vi "validate_experiment_pharmaBot_v0.06.vi"(0 "ExperimentOptionsCluster":T1, 1 "Open Tip?":bool, 4 "Graph cluster":T4, 7 "error in":errorcluster, 8 "which manipulator":T6(ring), 9 "common cluster":T8, 14 "controls array":refnum<vi>[](array[refnum]), 15 "individual controls in":T7, 17 "data in":T5={"daq_ao 1"="Dev1/ao0", "daq_ai 1"="Dev1/ai0", "experiment day folder"=path "D:/DATA/8-27-15 save func testing/test.lvm", "Multiclamp init error"=0, "Multiclamp Handle Out"=0, "sampling rate (Hz)"=10000, "trial name"=""}) -> (16 "control array out":refnum<vi>[](array[refnum]), 20 "ValidationWaveform":waveform(dbl)[](array[waveform]), 21 "protocol waveform":waveform(dbl)(graph), 22 "ValidationResults":waveform(dbl)[][](array[waveform]), 23 "ValidationPos1":T3(array[ring]), 24 "protocol response":waveform(dbl)[](graph), 25 "ValidationPos2":T3(array[ring]), 26 "ValidationOutputCluster":T2(array[cluster]), 27 "error out":errorcluster)   [LabVIEW 2019]
uses:
  pipette cleaning/pressure box/cleaning_soft/controls/actuator_type.ctl
  pipette cleaning/pressure box/cleaning_soft/controls/actuator_cluster.ctl
  machine_vision/coordinate model vis/transform_properties_actuators.ctl
  machine_vision/controls/transform_cluster_actuator.ctl
  controls/NH_method.ctl
  pipette cleaning/pressure box/cleaning_soft/controls/pressure_box_type.ctl
  pipette cleaning/pressure box/cleaning_soft/controls/pressure_box_control.ctl
  multipatch/controls/multipatch_common_controls_v4.ctl
  controls/memtest_def.ctl
  multipatch/controls/multipatch_individual_controls_v5.ctl
  Controls/Data.ctl
panel:
  out "curMJumpAlreadyValid":bool
  out "Jump Pos o-C":bool
  out "Jump Pos C-o":bool
  out "Jump Pos C-B":bool
  out "Jump Pos B-C":bool
  out "Jump Pos B-A":bool
  out "Jump Pos A-B":bool
  out "Jump Pos A-o":bool
  out "Jump Pos o-A":bool
  out "Pos C":bool
  out "Pos B":bool
  out "Pos A":bool
  out "Experiment Safe":bool
  out "Jumper Safe":bool
  # "already validated?"
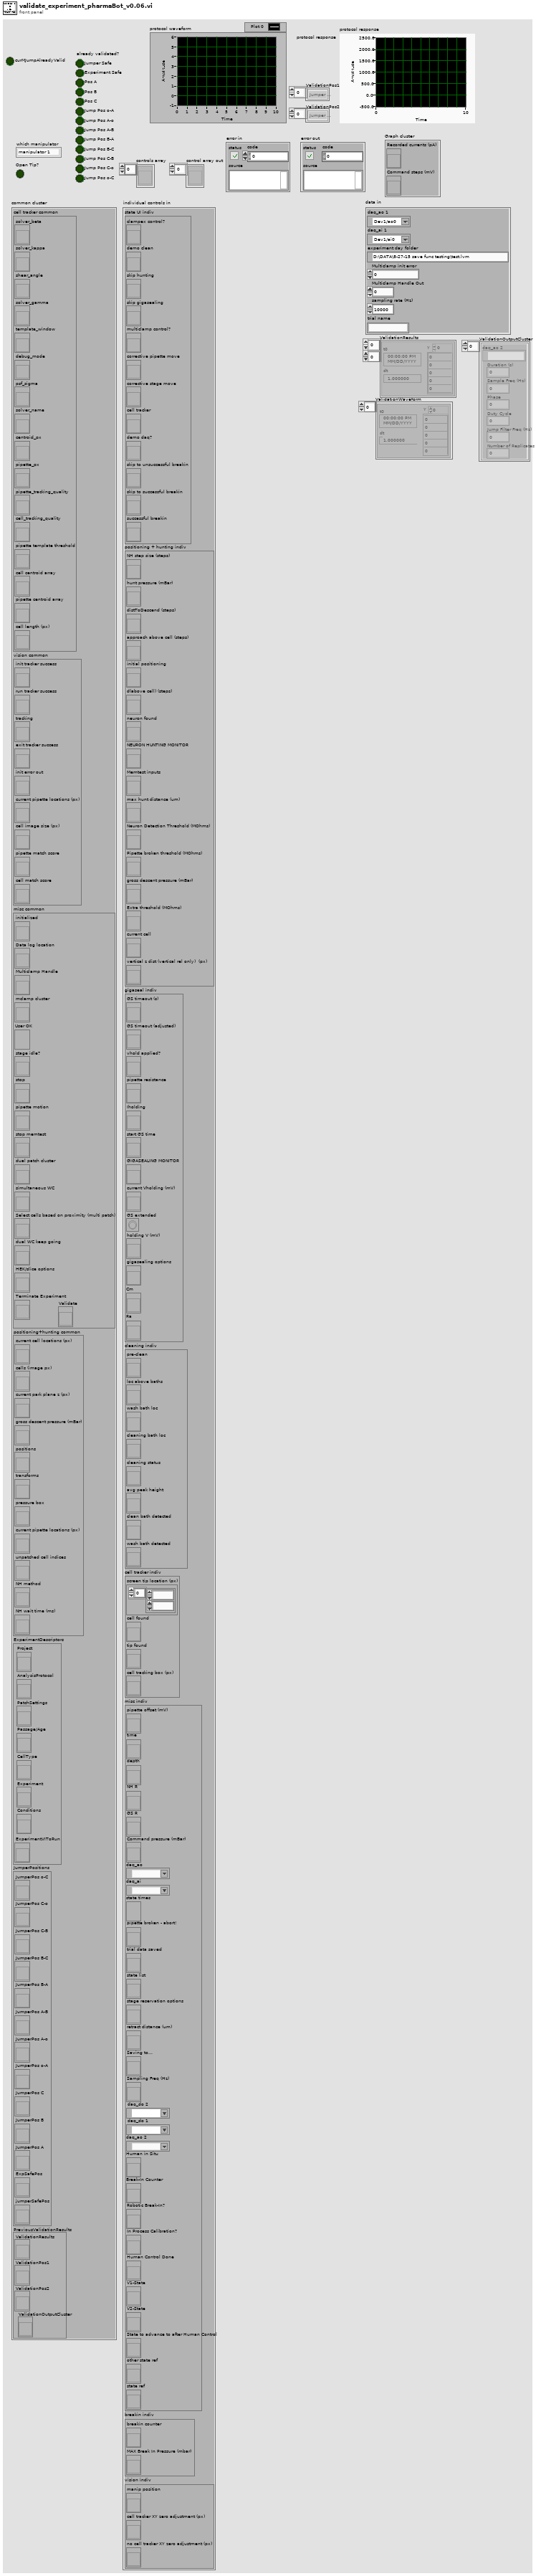
[diagram p1: front panel]
types:
  T1 = cluster{"How Many Experimental Phases?":refnum<vi>, "PhaseA Cluster":cluster{"Phase Experiment Option":refnum<vi>, "Paired Pulse":refnum<vi>, "Jump Train":refnum<vi>, "Voltage Ramp":refnum<vi>, "Voltage Step":refnum<vi>, "Solution Change":refnum<vi>, "Single Jump":refnum<vi>, "Single Manip Jump":refnum<vi>, "Gap Free":refnum<vi>, "Multi Manip Jump":refnum<vi>, "Voltage Pulse":refnum<vi>, "Current Pulse":refnum<vi>, "Current Ramp":refnum<vi>, "Gap Free Iclamp":refnum<vi>}, "PhaseB Cluster":cluster{"Phase Experiment Option":refnum<vi>, "Paired Pulse":refnum<vi>, "Jump Train":refnum<vi>, "Voltage Ramp":refnum<vi>, "Voltage Step":refnum<vi>, "Solution Change":refnum<vi>, "Single Jump":refnum<vi>, "Single Manip Jump":refnum<vi>, "Gap Free":refnum<vi>, "Multi Manip Jump":refnum<vi>, "Voltage Pulse":refnum<vi>, "Current Pulse":refnum<vi>, "Current Ramp":refnum<vi>, "Gap Free Iclamp":refnum<vi>}, "PhaseC Cluster":cluster{"Phase Experiment Option":refnum<vi>, "Paired Pulse":refnum<vi>, "Jump Train":refnum<vi>, "Voltage Ramp":refnum<vi>, "Voltage Step":refnum<vi>, "Solution Change":refnum<vi>, "Single Jump":refnum<vi>, "Single Manip Jump":refnum<vi>, "Gap Free":refnum<vi>, "Multi Manip Jump":refnum<vi>, "Voltage Pulse":refnum<vi>, "Current Pulse":refnum<vi>, "Current Ramp":refnum<vi>, "Gap Free Iclamp":refnum<vi>}, "PhaseD Cluster":cluster{"Phase Experiment Option":refnum<vi>, "Paired Pulse":refnum<vi>, "Jump Train":refnum<vi>, "Voltage Ramp":refnum<vi>, "Voltage Step":refnum<vi>, "Solution Change":refnum<vi>, "Single Jump":refnum<vi>, "Single Manip Jump":refnum<vi>, "Gap Free":refnum<vi>, "Multi Manip Jump":refnum<vi>, "Voltage Pulse":refnum<vi>, "Current Pulse":refnum<vi>, "Current Ramp":refnum<vi>, "Gap Free Iclamp":refnum<vi>}, "PhaseE Cluster":cluster{"Phase Experiment Option":refnum<vi>, "Paired Pulse":refnum<vi>, "Jump Train":refnum<vi>, "Voltage Ramp":refnum<vi>, "Voltage Step":refnum<vi>, "Solution Change":refnum<vi>, "Single Jump":refnum<vi>, "Single Manip Jump":refnum<vi>, "Gap Free":refnum<vi>, "Multi Manip Jump":refnum<vi>, "Voltage Pulse":refnum<vi>, "Current Pulse":refnum<vi>, "Current Ramp":refnum<vi>, "Gap Free Iclamp":refnum<vi>}, "PhaseF Cluster":cluster{"Phase Experiment Option":refnum<vi>, "Paired Pulse":refnum<vi>, "Jump Train":refnum<vi>, "Voltage Ramp":refnum<vi>, "Voltage Step":refnum<vi>, "Solution Change":refnum<vi>, "Single Jump":refnum<vi>, "Single Manip Jump":refnum<vi>, "Gap Free":refnum<vi>, "Multi Manip Jump":refnum<vi>, "Voltage Pulse":refnum<vi>, "Current Pulse":refnum<vi>, "Current Ramp":refnum<vi>, "Gap Free Iclamp":refnum<vi>}, "time to wait for solution change (min)":refnum<vi>, "valve Time Cluster":cluster{"time of Last V1 Change":refnum<vi>, "time of Last V2 Change":refnum<vi>, "time of Last V3 Change":refnum<vi>}, "PhaseG Cluster":cluster{"Phase Experiment Option":refnum<vi>, "Paired Pulse":refnum<vi>, "Jump Train":refnum<vi>, "Voltage Ramp":refnum<vi>, "Voltage Step":refnum<vi>, "Solution Change":refnum<vi>, "Single Jump":refnum<vi>, "Single Manip Jump":refnum<vi>, "Gap Free":refnum<vi>, "Multi Manip Jump":refnum<vi>, "Voltage Pulse":refnum<vi>, "Current Pulse":refnum<vi>, "Current Ramp":refnum<vi>, "Gap Free Iclamp":refnum<vi>}, "PhaseH Cluster":cluster{"Phase Experiment Option":refnum<vi>, "Paired Pulse":refnum<vi>, "Jump Train":refnum<vi>, "Voltage Ramp":refnum<vi>, "Voltage Step":refnum<vi>, "Solution Change":refnum<vi>, "Single Jump":refnum<vi>, "Single Manip Jump":refnum<vi>, "Gap Free":refnum<vi>, "Multi Manip Jump":refnum<vi>, "Voltage Pulse":refnum<vi>, "Current Pulse":refnum<vi>, "Current Ramp":refnum<vi>, "Gap Free Iclamp":refnum<vi>}, "PhaseI Cluster":cluster{"Phase Experiment Option":refnum<vi>, "Paired Pulse":refnum<vi>, "Jump Train":refnum<vi>, "Voltage Ramp":refnum<vi>, "Voltage Step":refnum<vi>, "Solution Change":refnum<vi>, "Single Jump":refnum<vi>, "Single Manip Jump":refnum<vi>, "Gap Free":refnum<vi>, "Multi Manip Jump":refnum<vi>, "Voltage Pulse":refnum<vi>, "Current Pulse":refnum<vi>, "Current Ramp":refnum<vi>, "Gap Free Iclamp":refnum<vi>}, "PhaseJ Cluster":cluster{"Phase Experiment Option":refnum<vi>, "Paired Pulse":refnum<vi>, "Jump Train":refnum<vi>, "Voltage Ramp":refnum<vi>, "Voltage Step":refnum<vi>, "Solution Change":refnum<vi>, "Single Jump":refnum<vi>, "Single Manip Jump":refnum<vi>, "Gap Free":refnum<vi>, "Multi Manip Jump":refnum<vi>, "Voltage Pulse":refnum<vi>, "Current Pulse":refnum<vi>, "Current Ramp":refnum<vi>, "Gap Free Iclamp":refnum<vi>}, "PhaseK Cluster":cluster{"Phase Experiment Option":refnum<vi>, "Paired Pulse":refnum<vi>, "Jump Train":refnum<vi>, "Voltage Ramp":refnum<vi>, "Voltage Step":refnum<vi>, "Solution Change":refnum<vi>, "Single Jump":refnum<vi>, "Single Manip Jump":refnum<vi>, "Gap Free":refnum<vi>, "Multi Manip Jump":refnum<vi>, "Voltage Pulse":refnum<vi>, "Current Pulse":refnum<vi>, "Current Ramp":refnum<vi>, "Gap Free Iclamp":refnum<vi>}, "PhaseL Cluster":cluster{"Phase Experiment Option":refnum<vi>, "Paired Pulse":refnum<vi>, "Jump Train":refnum<vi>, "Voltage Ramp":refnum<vi>, "Voltage Step":refnum<vi>, "Solution Change":refnum<vi>, "Single Jump":refnum<vi>, "Single Manip Jump":refnum<vi>, "Gap Free":refnum<vi>, "Multi Manip Jump":refnum<vi>, "Voltage Pulse":refnum<vi>, "Current Pulse":refnum<vi>, "Current Ramp":refnum<vi>, "Gap Free Iclamp":refnum<vi>}, "PhaseStatusCluster":cluster{"Phase A Done":refnum<vi>, "Phase B Done":refnum<vi>, "Phase C Done":refnum<vi>, "Phase D Done":refnum<vi>, "Phase E Done":refnum<vi>, "Phase F Done":refnum<vi>, "Phase G Done":refnum<vi>, "Phase H Done":refnum<vi>, "Phase I Done":refnum<vi>, "Phase J Done":refnum<vi>, "Phase K Done":refnum<vi>, "Phase L Done":refnum<vi>}}
  T2 = cluster{"daq_ao 2":tag, "Duration (s)":dbl, "Sample Freq (Hz)":dbl, "Phase":dbl, "Duty Cycle":dbl, "Jump Filter Freq (Hz)":dbl, "Number of Replicates":i16}[]
  T3 = enum16{"Jumper Safe Position", "Experiment Safe Position", "Jumper Position A", "Jumper Position B", "Jumper Position C", "Jumper Position o-A", "Jumper Position A-o", "Jumper Position A-B", "Jumper Position B-A", "Jumper Position B-C", "Jumper Position C-B", "Jumper Position C-o", "Jumper Position o-C"}[]
  T4 = cluster{"Recorded currents (pA)":refnum<vi>, "Command steps (mV)":refnum<vi>}
  T5 = typedef "Data.ctl" = cluster{"daq_ao 1":tag, "daq_ai 1":tag, "experiment day folder":path, "Multiclamp init error":i32, "Multiclamp Handle Out":u32, "sampling rate (Hz)":i32, "trial name":string}
  T6 = enum16{"manipulator 1", "manipulator 2", "manipulator 3", "manipulator 4"}
  T7 = typedef "multipatch_individual_controls_v5.ctl" = cluster{"state UI indiv":cluster{"clampex control?":refnum<vi>, "demo clean":refnum<vi>, "skip hunting":refnum<vi>, "skip gigasealing":refnum<vi>, "multiclamp control?":refnum<vi>, "corrective pipette move":refnum<vi>, "corrective stage move":refnum<vi>, "cell tracker":refnum<vi>, "demo daq?":refnum<vi>, "skip to unsuccessful breakin":refnum<vi>, "skip to successful breakin":refnum<vi>, "successful breakin":refnum<vi>}, "positioning + hunting indiv":cluster{"NH step size (steps)":refnum<vi>, "hunt pressure (mBar)":refnum<vi>, "distToDescend (steps)":refnum<vi>, "approach above cell (steps)":refnum<vi>, "initial positioning":refnum<vi>, "d(above cell) (steps)":refnum<vi>, "neuron found":refnum<vi>, "NEURON HUNTING MONITOR":refnum<vi>, "Memtest inputs":refnum<vi>, "max hunt distance (um)":refnum<vi>, "Neuron Detection Threshold (MOhms)":refnum<vi>, "Pipette broken threshold (MOhms)":refnum<vi>, "gross descent pressure (mBar)":refnum<vi>, "Extra threshold (MOhms)":refnum<vi>, "current cell":refnum<vi>, "vertical z dist (vertical rel only)  (px)":refnum<vi>}, "gigaseal indiv":cluster{"GS timeout (s)":refnum<vi>, "GS timeout (adjusted)":refnum<vi>, "vhold applied?":refnum<vi>, "pipette resistance":refnum<vi>, "Iholding":refnum<vi>, "start GS time":refnum<vi>, "GIGASEALING MONITOR":refnum<vi>, "current Vholding (mV)":refnum<vi>, "GS extended":refnum<vi>, "holding V (mV)":refnum<vi>, "gigasealing options":refnum<vi>, "Cm":refnum<vi>, "Ra ":refnum<vi>}, "cleaning indiv":cluster{"pre-clean":refnum<vi>, "loc above baths":refnum<vi>, "wash bath loc":refnum<vi>, "cleaning bath loc":refnum<vi>, "cleaning status":refnum<vi>, "avg peak height":refnum<vi>, "clean bath detected":refnum<vi>, "wash bath detected":refnum<vi>}, "cell tracker indiv":cluster{"screen tip location (px)":refnum<vi>, "cell found":refnum<vi>, "tip found":refnum<vi>, "cell tracking box (px)":refnum<vi>}, "misc indiv":cluster{"pipette offset (mV)":refnum<vi>, "time":refnum<vi>, "depth":refnum<vi>, "NH R":refnum<vi>, "GS R":refnum<vi>, "Command pressure (mBar)":refnum<vi>, "daq_ao":tag, "daq_ai":tag, "state times":refnum<vi>, "pipette broken - abort!":refnum<vi>, "trial data saved":refnum<vi>, "state list":refnum<vi>, "stage reservation options":refnum<vi>, "retract distance (um)":refnum<vi>, "Saving to...":refnum<vi>, "Sampling Freq (Hz)":refnum<vi>, "daq_do 2":tag, "daq_do 1":tag, "daq_ao 2":tag, "Human in Situ":refnum<vi>, "Break-In Counter":refnum<vi>, "Robotic Break-In?":refnum<vi>, "In Process Calibration?":refnum<vi>, "Human Control Done":refnum<vi>, "V1-State":refnum<vi>, "V2-State":refnum<vi>, "State to advance to after Human Control":refnum<vi>, "other state ref":refnum<vi>, "state ref":refnum<vi>}, "breakin indiv":cluster{"breakin counter":refnum<vi>, "MAX Break In Pressure (mbar)":refnum<vi>}, "vision indiv":cluster{"manip position":refnum<vi>, "cell tracker XY zero adjustment (px)":refnum<vi>, "no cell tracker XY zero adjustment (px)":refnum<vi>}}
  T8 = typedef "multipatch_common_controls_v4.ctl" = cluster{"cell tracker common":cluster{"solver_beta":refnum<vi>, "solver_kappa":refnum<vi>, "shear_angle":refnum<vi>, "solver_gamma":refnum<vi>, "template_window":refnum<vi>, "debug_mode":refnum<vi>, "psf_sigma":refnum<vi>, "solver_name":refnum<vi>, "centroid_px":refnum<vi>, "pipette_px":refnum<vi>, "pipette_tracking_quality":refnum<vi>, "cell_tracking_quality":refnum<vi>, "pipette template threshold":refnum<vi>, "cell centroid array":refnum<vi>, "pipette centroid array":refnum<vi>, "cell length (px)":refnum<vi>}, "vision common":cluster{"init tracker success":refnum<vi>, "run tracker success":refnum<vi>, "tracking":refnum<vi>, "exit tracker success":refnum<vi>, "init error out":refnum<vi>, "current pipette locations (px)":refnum<vi>, "cell image size (px)":refnum<vi>, "pipette match score":refnum<vi>, "cell match score":refnum<vi>}, "misc common":cluster{"initialized":refnum<vi>, "Data log location":refnum<vi>, "Multiclamp Handle":refnum<vi>, "mclamp cluster":refnum<vi>, "User OK":refnum<vi>, "stage idle?":refnum<vi>, "stop":refnum<vi>, "pipette motion":refnum<vi>, "stop memtest":refnum<vi>, "dual patch cluster":refnum<vi>, "simultaneous WC":refnum<vi>, "Select cells based on proximity (multi patch)":refnum<vi>, "dual WC keep going":refnum<vi>, "HEK/slice options":refnum<vi>, "Terminate Experiment":refnum<vi>, "Validate":refnum<vi>}, "positioning+hunting common":cluster{"current cell locations (px)":refnum<vi>, "cells (image px)":refnum<vi>, "current park plane z (px)":refnum<vi>, "gross descent pressure (mBar)":refnum<vi>, "positions":refnum<vi>, "transforms":refnum<vi>, "pressure box":refnum<vi>, "current pipette locations (px)":refnum<vi>, "unpatched cell indices":refnum<vi>, "NH method":refnum<vi>, "NH wait time (ms)":refnum<vi>}, "ExperimentDescriptors":cluster{"Project":refnum<vi>, "AnalysisProtocol":refnum<vi>, "PatchSettings":refnum<vi>, "Passage/Age":refnum<vi>, "CellType":refnum<vi>, "Experiment":refnum<vi>, "Conditions":refnum<vi>, "ExperimentVIToRun":refnum<vi>}, "JumperPositions":cluster{"JumperPos o-C":refnum<vi>, "JumperPos C-o":refnum<vi>, "JumperPos C-B":refnum<vi>, "JumperPos B-C":refnum<vi>, "JumperPos B-A":refnum<vi>, "JumperPos A-B":refnum<vi>, "JumperPos A-o":refnum<vi>, "JumperPos o-A":refnum<vi>, "JumperPos C":refnum<vi>, "JumperPos B":refnum<vi>, "JumperPos A":refnum<vi>, "ExpSafePos":refnum<vi>, "jumperSafePos":refnum<vi>}, "PreviousValidationResults":cluster{"ValidationResults":refnum<vi>, "ValidationPos1":refnum<vi>, "ValidationPos2":refnum<vi>, "ValidationOutputCluster":refnum<vi>}}
  T9 = cluster{"time of Last V1 Change":refnum<vi>, "time of Last V2 Change":refnum<vi>, "time of Last V3 Change":refnum<vi>}
  T10 = typedef "pressure_box_control.ctl" = cluster{"Pressure box COM":refnum<visa-resource-name>, "pressure box type":T11, "High pos pressure (mBar)":dbl, "Low pos pressure (mBar)":dbl, "Vacuum pressure (mBar)":dbl, "calibration":enum16{"PA_vacPump", "PA_venturi", "Neuromatics", "ilyaRig", "mightenRig"}}
  T11 = typedef "pressure_box_type.ctl" = enum16{"Neuromatics", "ProportionAir", "Demo box", "N-ProportionAir"}
  T12 = cluster{"daq_ao 2":tag, "Duration (s)":dbl, "Sample Freq (Hz)":dbl, "Phase":dbl, "Duty Cycle":dbl, "Jump Filter Freq (Hz)":dbl, "Number of Replicates":i16}
  T13 = enum16{"Jumper Safe Position", "Experiment Safe Position", "Jumper Position A", "Jumper Position B", "Jumper Position C", "Jumper Position o-A", "Jumper Position A-o", "Jumper Position A-B", "Jumper Position B-A", "Jumper Position B-C", "Jumper Position C-B", "Jumper Position C-o", "Jumper Position o-C"}
  T14 = cluster{u32, string, i32, u32, u32, u32, "arg1":i32}
  T15 = cluster{"Phase Experiment Option":refnum<vi>, "Paired Pulse":refnum<vi>, "Jump Train":refnum<vi>, "Voltage Ramp":refnum<vi>, "Voltage Step":refnum<vi>, "Solution Change":refnum<vi>, "Single Jump":refnum<vi>, "Single Manip Jump":refnum<vi>, "Gap Free":refnum<vi>, "Multi Manip Jump":refnum<vi>, "Voltage Pulse":refnum<vi>, "Current Pulse":refnum<vi>, "Current Ramp":refnum<vi>, "Gap Free Iclamp":refnum<vi>}
  T16 = cluster{"Which Position to use for Experiment":enum16{"Jumper Safe Position", "Experiment Safe Position", "Jumper Position A", "Jumper Position B", "Jumper Position C", "Jumper Position o-A", "Jumper Position A-o", "Jumper Position A-B", "Jumper Position B-A", "Jumper Position B-C", "Jumper Position C-B", "Jumper Position C-o", "Jumper Position o-C", "Don't Move"}, "Start Position (N)":string, "Jump Position (m)":string, "Duration (s)":dbl, "Delay (s)":dbl, "Pulse Width (s)":dbl, "Valve 1 Position":i16, "Valve 2 Position":i16, "Replicates":dbl, "Vholding (mV)":dbl, "Valve 3 Position":i16, "valve 1 used now?":bool, "valve 2 used now?":bool, "valve 3 used now? ":bool, "protocol Preview":waveform(dbl)[]}
  T17 = enum16{"Jumper Safe Position", "Experiment Safe Position", "Jumper Position A", "Jumper Position B", "Jumper Position C", "Jumper Position o-A", "Jumper Position A-o", "Jumper Position A-B", "Jumper Position B-A", "Jumper Position B-C", "Jumper Position C-B", "Jumper Position C-o", "Jumper Position o-C", "Don't Move"}
  T18 = cluster{"Which Position to use for Experiment":enum16{"Jumper Safe Position", "Experiment Safe Position", "Jumper Position A", "Jumper Position B", "Jumper Position C", "Jumper Position o-A", "Jumper Position A-o", "Jumper Position A-B", "Jumper Position B-A", "Jumper Position B-C", "Jumper Position C-B", "Jumper Position C-o", "Jumper Position o-C", "Don't Move"}, "Duration (s)":dbl, "Delay (s)":dbl, "Pulse Width (s)":dbl, "Which Valve to Change?":i16, "Valve Jump Position":i16, "Replicates":dbl, "Vholding (mV)":dbl, "valve 1 used now?":bool, "valve 2 used now?":bool, "valve 3 used now? ":bool, "Valve 1 Position":i16, "Valve 2 Position":i16, "Valve 3 Position":i16, "protocol Preview":waveform(dbl)[]}
  T19 = cluster{"Which Position to use for Experiment":enum16{"Jumper Safe Position", "Experiment Safe Position", "Jumper Position A", "Jumper Position B", "Jumper Position C", "Jumper Position o-A", "Jumper Position A-o", "Jumper Position A-B", "Jumper Position B-A", "Jumper Position B-C", "Jumper Position C-B", "Jumper Position C-o", "Jumper Position o-C", "Don't Move"}, "Duration (s)":dbl, "Delay (s)":dbl, "Step Width (s)":dbl, "Voltage Start (mV)":dbl, "Voltage Step (mV)":dbl, "Replicates":dbl, "Voltage End (mV)":dbl, "Number of Step":dbl, "Vholding (mV)":dbl, "Valve 1 Position":i16, "Valve 2 Position":i16, "Valve 3 Position":i16, "valve 1 used now?":bool, "valve 2 used now?":bool, "valve 3 used now? ":bool, "Total Step Time (s)":dbl, "Maintain Final Voltage until end?":bool, "protocol Preview":waveform(dbl)[]}
  T20 = cluster{"Which Position to use for Experiment":enum16{"Jumper Safe Position", "Experiment Safe Position", "Jumper Position A", "Jumper Position B", "Jumper Position C", "Jumper Position o-A", "Jumper Position A-o", "Jumper Position A-B", "Jumper Position B-A", "Jumper Position B-C", "Jumper Position C-B", "Jumper Position C-o", "Jumper Position o-C", "Don't Move"}, "Duration (s)":dbl, "Delay (s)":dbl, "Ramp Slope (mV/s)":dbl, "Voltage Start (mV)":dbl, "Replicates":dbl, "Voltage End (mV)":dbl, "Ramp Duration (s)":dbl, "Vholding (mV)":dbl, "Valve 1 Position":i16, "Valve 2 Position":i16, "Valve 3 Position":i16, "valve 1 used now?":bool, "valve 2 used now?":bool, "valve 3 used now? ":bool, "Maintain Final Voltage until end?":bool, "protocol Preview":waveform(dbl)[]}
  T21 = cluster{"Which Position to use for Experiment":enum16{"Jumper Safe Position", "Experiment Safe Position", "Jumper Position A", "Jumper Position B", "Jumper Position C", "Jumper Position o-A", "Jumper Position A-o", "Jumper Position A-B", "Jumper Position B-A", "Jumper Position B-C", "Jumper Position C-B", "Jumper Position C-o", "Jumper Position o-C", "Don't Move"}, "Start Position (N)":string, "Jump Position (m)":string, "Duration (s)":dbl, "Delay (s)":dbl, "Pulse Width (s)":dbl, "Valve 1 Position":i16, "Valve 2 Position":i16, "Replicates":dbl, "Pulse Period (s)":dbl, "Vholding (mV)":dbl, "Number of Pulses":dbl, "valve 1 used now?":bool, "valve 2 used now?":bool, "valve 3 used now? ":bool, "Valve 3 Position":i16, "protocol Preview":waveform(dbl)[]}
  T22 = cluster{"Which Position to use for Experiment":enum16{"Jumper Safe Position", "Experiment Safe Position", "Jumper Position A", "Jumper Position B", "Jumper Position C", "Jumper Position o-A", "Jumper Position A-o", "Jumper Position A-B", "Jumper Position B-A", "Jumper Position B-C", "Jumper Position C-B", "Jumper Position C-o", "Jumper Position o-C", "Don't Move"}, "Start Position (N)":string, "Jump Position (m)":string, "Duration (s)":dbl, "Delay (s)":dbl, "Pulse Width (s)":dbl, "Replicates":dbl, "Pulse Delay (s)":dbl, "Pulse Delta Delay (s)":dbl, "Vholding (mV)":dbl, "Valve 1 Position":i16, "Valve 2 Position":i16, "valve 1 used now?":bool, "valve 2 used now?":bool, "valve 3 used now? ":bool, "Valve 3 Position":i16, "protocol Preview":waveform(dbl)[]}
  T23 = cluster{"Start Position (N)":enum16{"Jumper Safe Position", "Experiment Safe Position", "Jumper Position A", "Jumper Position B", "Jumper Position C", "Jumper Position o-A", "Jumper Position A-o", "Jumper Position A-B", "Jumper Position B-A", "Jumper Position B-C", "Jumper Position C-B", "Jumper Position C-o", "Jumper Position o-C", "Don't Move"}, "Duration (s)":dbl, "Delay (s)":dbl, "Pulse Width (s)":dbl, "Valve 1 Position":i16, "Valve 2 Position":i16, "Replicates":dbl, "Jump Position (m)":enum16{"Jumper Safe Position", "Experiment Safe Position", "Jumper Position A", "Jumper Position B", "Jumper Position C", "Jumper Position o-A", "Jumper Position A-o", "Jumper Position A-B", "Jumper Position B-A", "Jumper Position B-C", "Jumper Position C-B", "Jumper Position C-o", "Jumper Position o-C", "Don't Move"}, "Vholding (mV)":dbl, "Valve 3 Position":i16, "valve 1 used now?":bool, "valve 2 used now?":bool, "valve 3 used now? ":bool, "protocol Preview":waveform(dbl)[]}
  T24 = enum16{"Jumper Safe Position", "Experiment Safe Position", "Jumper Position A", "Jumper Position B", "Jumper Position C", "Jumper Position o-A", "Jumper Position A-o", "Jumper Position A-B", "Jumper Position B-A", "Jumper Position B-C", "Jumper Position C-B", "Jumper Position C-o", "Jumper Position o-C", "Don't Move"}[]
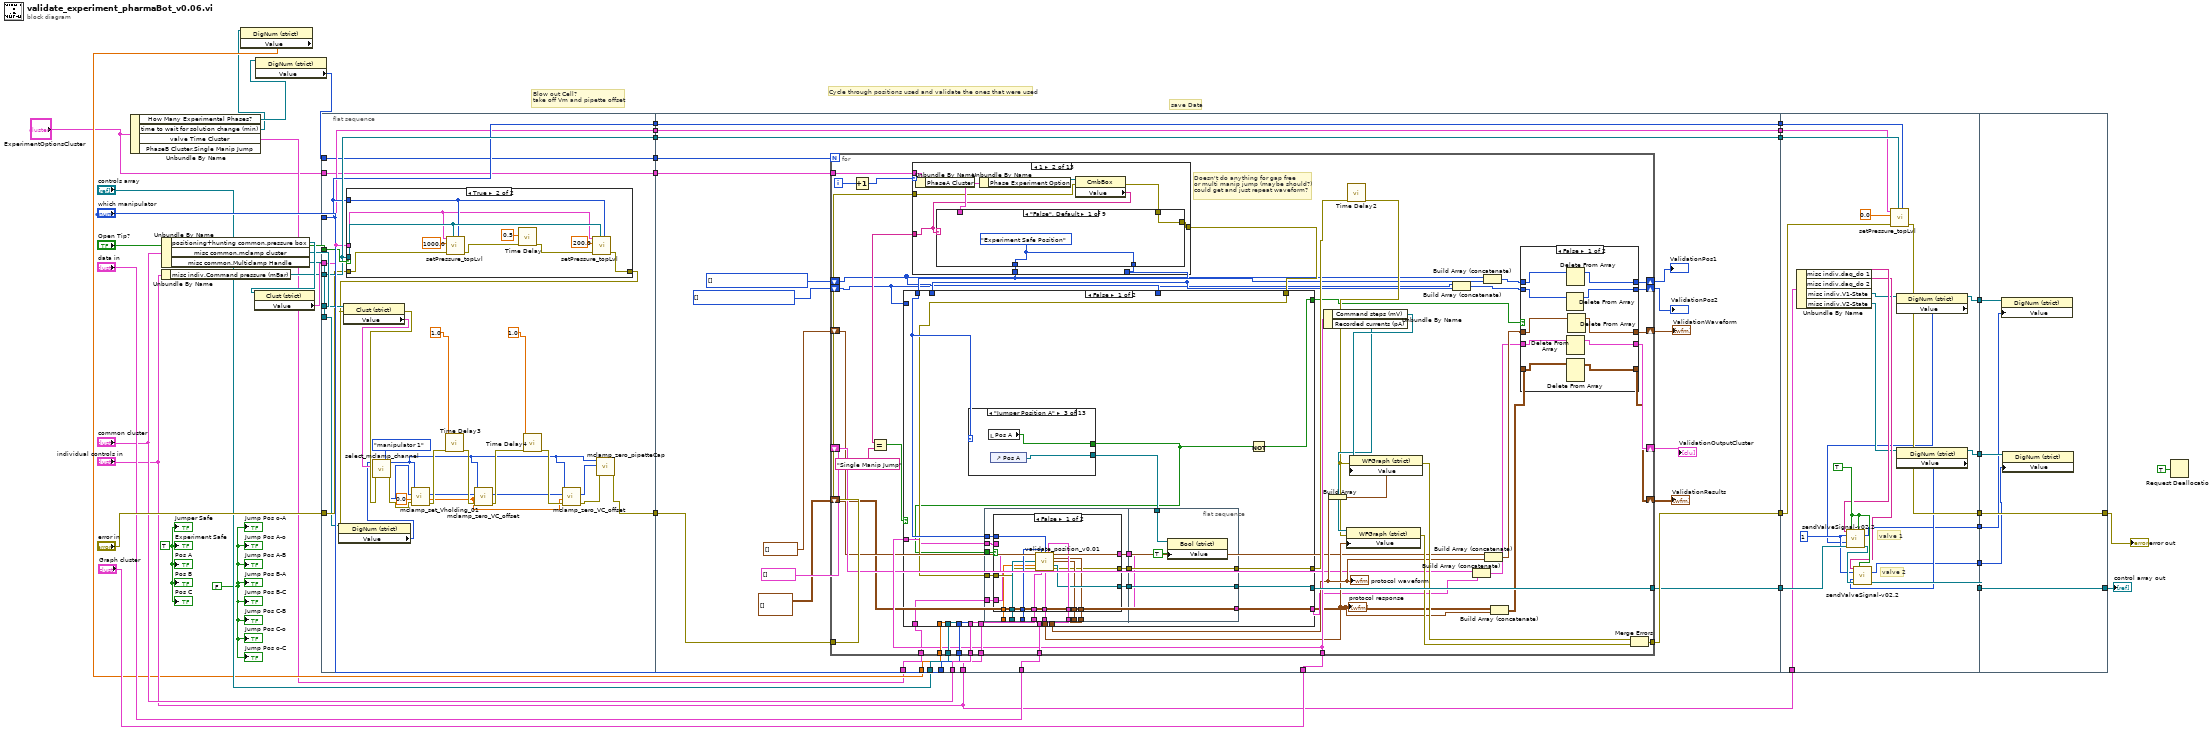
[diagram p0: block diagram]
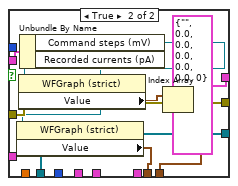
[diagram p4: hidden frame]
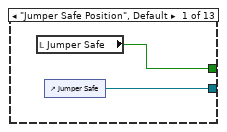
[diagram p5: hidden frame]
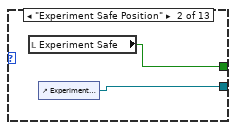
[diagram p6: hidden frame]
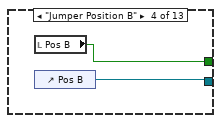
[diagram p7: hidden frame]
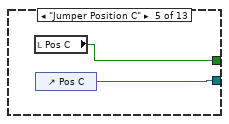
[diagram p8: hidden frame]
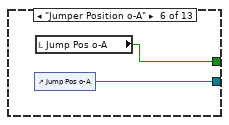
[diagram p9: hidden frame]
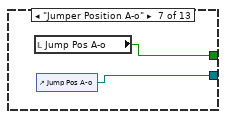
[diagram p10: hidden frame]
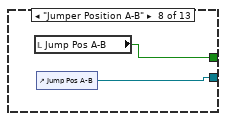
[diagram p11: hidden frame]
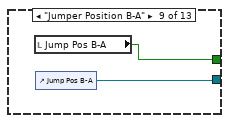
[diagram p12: hidden frame]
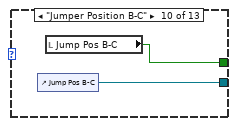
[diagram p13: hidden frame]
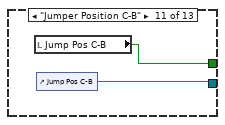
[diagram p14: hidden frame]
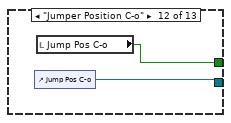
[diagram p15: hidden frame]
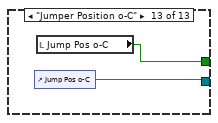
[diagram p16: hidden frame]
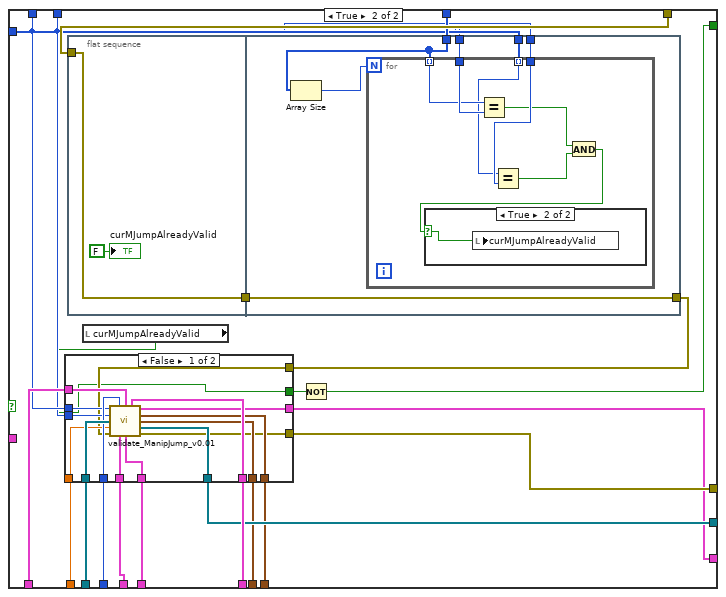
[diagram p17: hidden frame]
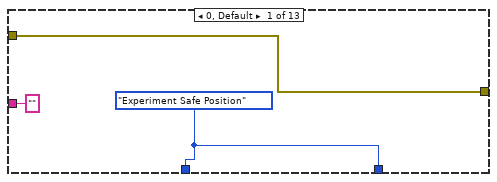
[diagram p20: hidden frame]
diagram:
  w18 = FALSE
  w20 = TRUE ("Experiment Safe")
  # "save Data"
  # "Cycle through positions used and validate the ones that were used"
  # "Blow out Cell?\ntake off Vm and pipette offset"
  n1 = Unbundle By Name("ExperimentOptionsCluster") -> ("How Many Experimental Phases?"=w28:refnum<vi>, "time to wait for solution change (min)"=w4:refnum<vi>, "valve Time Cluster"=w3:T9)  [unwired: 1 out]
  n2 = Unbundle By Name("individual controls in") -> ("misc indiv.Command pressure (mBar)"=w36:refnum<vi>)
  n3 = Unbundle By Name("common cluster") -> ("positioning+hunting common.pressure box"=w38:refnum<vi>, "misc common.mclamp cluster"=w7:refnum<vi>, "misc common.Multiclamp Handle"=w6:refnum<vi>)
  n4 = property class="DigNum (strict)"(reference=w4) -> ("Value"=w5:dbl)  [unwired: 1 in, 2 out]
  n5 = property class="Clust (strict)"(reference=w38) -> ("Value"=w37:T10)  [unwired: 1 in, 2 out]
  n6 = property class="DigNum (strict)"(reference=w28) -> ("Value"=w27:i32)  [unwired: 1 in, 2 out]
  n7 = flat-sequence {
    tunnel: "error in" -> [w50]
    tunnel: [w44] -> w40
    tunnel: "which manipulator" -> [w68]
    tunnel: w37 -> [w67]
    tunnel: w36 -> [w69]
    tunnel: "Open Tip?" -> [w70]
    tunnel: [w69] -> w34
    tunnel: [w68] -> w32
    tunnel: [w67] -> w30
    tunnel: w27 -> [w66]
    tunnel: [w66] -> w26
    tunnel: "ExperimentOptionsCluster" -> [w65]
    tunnel: [w65] -> w25
    tunnel: w7 -> [w51]
    tunnel: w6 -> [w49]
    tunnel: w40 -> [w102]
    tunnel: w34 -> [w107]
    tunnel: [w107] -> w33
    tunnel: w32 -> [w106]
    tunnel: [w106] -> w31
    tunnel: w30 -> [w105]
    tunnel: [w105] -> w29
    tunnel: w26 -> [w104]
    tunnel: w25 -> [w103]
    tunnel: [w101] -> w24
    tunnel: "common cluster" -> [w100]
    tunnel: "individual controls in" -> [w99]
    tunnel: "which manipulator" -> [w98]
    tunnel: "data in" -> [w97]
    tunnel: "controls array" -> [w96]
    tunnel: [w95] -> w19
    tunnel: "Graph cluster" -> [w94]
    tunnel: w5 -> [w93]
    tunnel: w3 -> [w92]
    tunnel: w33 -> [w1084]
    tunnel: w31 -> [w1083]
    tunnel: w29 -> [w1082]
    tunnel: w24 -> [w1081]
    tunnel: w19 -> [w1078]
    tunnel: "individual controls in" -> [w1074]
    tunnel: [w1080] -> w13
    tunnel: [w1077] -> w12
    tunnel: [w1069] -> w11
    tunnel: [w1068] -> w10
    tunnel: [w1065] -> w9
    tunnel: [w1064] -> w8
    tunnel: [w1090] -> w17
    tunnel: [w1091] -> w39
    tunnel: w13 -> [w1091]
    tunnel: w12 -> [w1090]
    tunnel: w11 -> [w1089]
    tunnel: w10 -> [w1088]
    tunnel: w9 -> [w1087]
    tunnel: w8 -> [w1086]
    frame #0 {
      w46 = 0.0 ("set holding (mV)")
      n8 = case shown="True" w70 {
        tunnel: w50 -> [w71 w80]
        tunnel: [w71 w77] -> w47
        tunnel: w68 -> [_ w73]
        tunnel: w67 -> [_ w72]
        tunnel: w69 -> [_ w74]
        frame False {
        }
        frame True {
          n9 = call "setPressure_topLvl.vi"("which manipulator"=w73, "Slide Refnum"=w74, "error in"=w80, "set pressure (mBar)"=1000.0, "Pressure box control in"=w72) -> ("error out"=w79:errorcluster)  [unwired: 5 in, 1 out]
          n10 = call "Time Delay"("error in (no error)"=w79, "Delay Time (s)"=0.5) -> ("error out"=w78:errorcluster)  [unwired: 9 in]
          n11 = call "setPressure_topLvl.vi"("which manipulator"=w73, "Slide Refnum"=w74, "error in"=w78, "set pressure (mBar)"=200.0, "Pressure box control in"=w72) -> ("error out"=w77:errorcluster)  [unwired: 5 in, 1 out]
        }
      }
      n12 = property class="DigNum (strict)"(reference=w49, error in=w47) -> ("Value"=w48:u32)  [unwired: 2 out]
      n13 = property class="Clust (strict)"(reference=w51, error in=w47) -> (error out=w56:errorcluster, "Value"=w53:T14)  [unwired: 1 out]
      n14 = call "select_mclamp_channel.vi"("which manipulator"=T6."manipulator 1", "error in (no error)"=w56, "mclamp cluster"=w53, "Multiclamp Handle In"=w48) -> ("error out"=w55:errorcluster, "error"=w54:i32, "Multiclamp Handle out"=w43:u32)  [unwired: 5 in]
      n15 = call "mclamp_set_Vholding_01.vi"("error in (no error)"=w55, "set holding (mV)"=w46, "Error in"=w54, "Multiclamp Handle Out"=w43) -> (0:"error out"=w62:errorcluster, 2:"error out"=w58:i32)  [unwired: 6 in]
      n16 = call "Time Delay3"("error in (no error)"=w62, "Delay Time (s)"=1.0) -> ("error out"=w61:errorcluster)  [unwired: 9 in]
      n17 = call "mclamp_zero_VC_offset.vi"("error in (no error)"=w61, "set holding (mV)"=w46, "Error in"=w58, "Multiclamp Handle Out"=w43) -> (0:"error out"=w60:errorcluster, 2:"error out"=w57:i32)  [unwired: 6 in]
      n18 = call "Time Delay4"("error in (no error)"=w60, "Delay Time (s)"=1.0) -> ("error out"=w59:errorcluster)  [unwired: 9 in]
      n19 = call "mclamp_zero_VC_offset.vi"("error in (no error)"=w59, "set holding (mV)"=w46, "Error in"=w57, "Multiclamp Handle Out"=w43) -> (0:"error out"=w45:errorcluster, 2:"error out"=w42:i32)  [unwired: 6 in]
      n20 = call "mclamp_zero_pipetteCap.vi"("error in (no error)"=w45, "Error in"=w42, "Multiclamp Handle Out"=w43) -> ("error out"=w44:errorcluster)  [unwired: 6 in, 2 out]
    }
    frame #1 {
      w85 = T3 [] items=["Jumper Safe Position", "Experiment Safe Position", "Jumper Position A", "Jumper Position B", "Jumper Position C", "Jumper Position o-A", "Jumper Position A-o", "Jumper Position A-B", "Jumper Position B-A", "Jumper Position B-C", "Jumper Position C-B", "Jumper Position C-o", "Jumper Position o-C"]
      w86 = T3 [] items=["Jumper Safe Position", "Experiment Safe Position", "Jumper Position A", "Jumper Position B", "Jumper Position C", "Jumper Position o-A", "Jumper Position A-o", "Jumper Position A-B", "Jumper Position B-A", "Jumper Position B-C", "Jumper Position C-B", "Jumper Position C-o", "Jumper Position o-C"]
      n21 = for {
        N: w104 -> [_]
        tunnel: w103 -> [w152]
        tunnel: w102 -> [w138]
        tunnel: [w133] -> w101
        tunnel: w100 -> [w151]
        tunnel: w99 -> [w150]
        tunnel: w98 -> [w149]
        tunnel: w97 -> [w148]
        tunnel: w96 -> [w147]
        tunnel: [w142] -> w95
        tunnel: w94 -> [w130]
        tunnel: w93 -> [w131]
        tunnel: w92 -> [w129]
        shift-right: [w114] -> w91
        shift-left: w86 -> [w109]
        shift-right: [w113] -> w90
        shift-left: w85 -> [w108]
        shift-right: [w112] -> w89
        shift-left: waveform(dbl)[] [] -> [w122]
        shift-right: [w110] -> w88
        shift-left: waveform(dbl)[][] [] -> [w121]
        shift-right: [w111] -> w87
        shift-left: T2 [] -> [w123]
        i -> [w153]
        # "Doesn't do anything for gap free\nor multi manip jump (maybe should?)\ncould get and just repeat waveform?"
        n22 = Increment(x=w153) -> (x+1=w143:i32)
        n23 = case shown="1" w143 {
          tunnel: w152 -> [_ w328 w390 w452 w514 w576 w638 w700 w762 w824 w886 w948 w1010]
          tunnel: [w319 w326 w388 w450 w512 w574 w636 w698 w760 w822 w884 w946 w1008] -> w128
          tunnel: [w319 w324 w386 w448 w510 w572 w634 w696 w758 w820 w882 w944 w1006] -> w127
          tunnel: ["" ("Value") w323 w385 w447 w509 w571 w633 w695 w757 w819 w881 w943 w1005] -> w146
          tunnel: w138 -> [w317 w322 w384 w446 w508 w570 w632 w694 w756 w818 w880 w942 w1004]
          tunnel: [w317 w320 w382 w444 w506 w568 w630 w692 w754 w816 w878 w940 w1002] -> w137
          frame 0, Default {
            w319 = T13."Experiment Safe Position" ("Which Position to use for Experiment")
          }
          frame 1 {
            n24 = Unbundle By Name(w328) -> ("PhaseA Cluster"=w325:T15)
            n25 = Unbundle By Name(w325) -> ("Phase Experiment Option"=w327:refnum<vi>)
            n26 = property class="CmbBox"(reference=w327, error in=w322) -> (error out=w321:errorcluster, "Value"=w323:string)  [unwired: 1 out]
            n27 = case shown="\"False\", Default" w323 {
              tunnel: w325 -> [_ w337 w343 w349 w356 w363 w370 w378 _]
              tunnel: [w330 w334 w341 w348 w355 w362 w369 w377 w381] -> w326
              tunnel: [w330 T13."Experiment Safe Position" ("Which Position to use for Experiment") T13."Experiment Safe Position" ("Which Position to use for Experiment") T13."Experiment Safe Position" ("Which Position to use for Experiment") T13."Experiment Safe Position" ("Which Position to use for Experiment") T13."Experiment Safe Position" ("Which Position to use for Experiment") T13."Experiment Safe Position" ("Which Position to use for Experiment") w375 w381] -> w324
              tunnel: w321 -> [w329 w332 w339 w346 w353 w360 w367 w374 w380]
              tunnel: [w329 w331 w338 w345 w352 w359 w366 w373 w380] -> w320
              frame "False", Default {
                w330 = T13."Experiment Safe Position" ("Which Position to use for Experiment")
              }
              frame "Single Jump" {
                n28 = Unbundle By Name(w337) -> ("Single Jump"=w336:refnum<vi>)
                n29 = property class="Clust (strict)"(reference=w336, error in=w332) -> (error out=w331:errorcluster, "Value"=w335:T16)  [unwired: 1 out]
                n30 = Unbundle By Name(w335) -> ("Which Position to use for Experiment"=w334:T17)
              }
              frame "Solution Change" {
                n31 = Unbundle By Name(w343) -> ("Solution Change"=w344:refnum<vi>)
                n32 = property class="Clust (strict)"(reference=w344, error in=w339) -> (error out=w338:errorcluster, "Value"=w342:T18)  [unwired: 1 out]
                n33 = Unbundle By Name(w342) -> ("Which Position to use for Experiment"=w341:T17)
              }
              frame "Voltage Step" {
                n34 = Unbundle By Name(w349) -> ("Voltage Step"=w351:refnum<vi>)
                n35 = property class="Clust (strict)"(reference=w351, error in=w346) -> (error out=w345:errorcluster, "Value"=w350:T19)  [unwired: 1 out]
                n36 = Unbundle By Name(w350) -> ("Which Position to use for Experiment"=w348:T17)
              }
              frame "Voltage Ramp" {
                n37 = Unbundle By Name(w356) -> ("Voltage Ramp"=w358:refnum<vi>)
                n38 = property class="Clust (strict)"(reference=w358, error in=w353) -> (error out=w352:errorcluster, "Value"=w357:T20)  [unwired: 1 out]
                n39 = Unbundle By Name(w357) -> ("Which Position to use for Experiment"=w355:T17)
              }
              frame "Jump Train" {
                n40 = Unbundle By Name(w363) -> ("Jump Train"=w365:refnum<vi>)
                n41 = property class="Clust (strict)"(reference=w365, error in=w360) -> (error out=w359:errorcluster, "Value"=w364:T21)  [unwired: 1 out]
                n42 = Unbundle By Name(w364) -> ("Which Position to use for Experiment"=w362:T17)
              }
              frame "Paired Pulse" {
                n43 = Unbundle By Name(w370) -> ("Paired Pulse"=w372:refnum<vi>)
                n44 = property class="Clust (strict)"(reference=w372, error in=w367) -> (error out=w366:errorcluster, "Value"=w371:T22)  [unwired: 1 out]
                n45 = Unbundle By Name(w371) -> ("Which Position to use for Experiment"=w369:T17)
              }
              frame "Single Manip Jump" {
                n46 = Unbundle By Name(w378) -> ("Single Manip Jump"=w379:refnum<vi>)
                n47 = property class="Clust (strict)"(reference=w379, error in=w374) -> (error out=w373:errorcluster, "Value"=w376:T23)  [unwired: 1 out]
                n48 = Unbundle By Name(w376) -> ("Start Position (N)"=w377:T17)
                n49 = Unbundle By Name(w376) -> ("Jump Position (m)"=w375:T17)
              }
              frame "none" {
                w381 = T13."Experiment Safe Position" ("Which Position to use for Experiment")
              }
            }
          }
          frame 2 {
            n50 = Unbundle By Name(w390) -> ("PhaseB Cluster"=w387:T15)
            n51 = Unbundle By Name(w387) -> ("Phase Experiment Option"=w389:refnum<vi>)
            n52 = property class="CmbBox"(reference=w389, error in=w384) -> (error out=w383:errorcluster, "Value"=w385:string)  [unwired: 1 out]
            n53 = case shown="\"Single Manip Jump\"" w385 {
              tunnel: w387 -> [_ w399 w405 w411 w418 w425 w432 w440 _]
              tunnel: [w392 w396 w403 w410 w417 w424 w431 w439 w443] -> w388
              tunnel: [w392 T13."Experiment Safe Position" ("Which Position to use for Experiment") T13."Experiment Safe Position" ("Which Position to use for Experiment") T13."Experiment Safe Position" ("Which Position to use for Experiment") T13."Experiment Safe Position" ("Which Position to use for Experiment") T13."Experiment Safe Position" ("Which Position to use for Experiment") T13."Experiment Safe Position" ("Which Position to use for Experiment") w437 w443] -> w386
              tunnel: w383 -> [w391 w394 w401 w408 w415 w422 w429 w436 w442]
              tunnel: [w391 w393 w400 w407 w414 w421 w428 w435 w442] -> w382
              frame "False", Default {
                w392 = T13."Experiment Safe Position" ("Which Position to use for Experiment")
              }
              frame "Single Jump" {
                n54 = Unbundle By Name(w399) -> ("Single Jump"=w398:refnum<vi>)
                n55 = property class="Clust (strict)"(reference=w398, error in=w394) -> (error out=w393:errorcluster, "Value"=w397:T16)  [unwired: 1 out]
                n56 = Unbundle By Name(w397) -> ("Which Position to use for Experiment"=w396:T17)
              }
              frame "Solution Change" {
                n57 = Unbundle By Name(w405) -> ("Solution Change"=w406:refnum<vi>)
                n58 = property class="Clust (strict)"(reference=w406, error in=w401) -> (error out=w400:errorcluster, "Value"=w404:T18)  [unwired: 1 out]
                n59 = Unbundle By Name(w404) -> ("Which Position to use for Experiment"=w403:T17)
              }
              frame "Voltage Step" {
                n60 = Unbundle By Name(w411) -> ("Voltage Step"=w413:refnum<vi>)
                n61 = property class="Clust (strict)"(reference=w413, error in=w408) -> (error out=w407:errorcluster, "Value"=w412:T19)  [unwired: 1 out]
                n62 = Unbundle By Name(w412) -> ("Which Position to use for Experiment"=w410:T17)
              }
              frame "Voltage Ramp" {
                n63 = Unbundle By Name(w418) -> ("Voltage Ramp"=w420:refnum<vi>)
                n64 = property class="Clust (strict)"(reference=w420, error in=w415) -> (error out=w414:errorcluster, "Value"=w419:T20)  [unwired: 1 out]
                n65 = Unbundle By Name(w419) -> ("Which Position to use for Experiment"=w417:T17)
              }
              frame "Jump Train" {
                n66 = Unbundle By Name(w425) -> ("Jump Train"=w427:refnum<vi>)
                n67 = property class="Clust (strict)"(reference=w427, error in=w422) -> (error out=w421:errorcluster, "Value"=w426:T21)  [unwired: 1 out]
                n68 = Unbundle By Name(w426) -> ("Which Position to use for Experiment"=w424:T17)
              }
              frame "Paired Pulse" {
                n69 = Unbundle By Name(w432) -> ("Paired Pulse"=w434:refnum<vi>)
                n70 = property class="Clust (strict)"(reference=w434, error in=w429) -> (error out=w428:errorcluster, "Value"=w433:T22)  [unwired: 1 out]
                n71 = Unbundle By Name(w433) -> ("Which Position to use for Experiment"=w431:T17)
              }
              frame "Single Manip Jump" {
                n72 = Unbundle By Name(w440) -> ("Single Manip Jump"=w441:refnum<vi>)
                n73 = property class="Clust (strict)"(reference=w441, error in=w436) -> (error out=w435:errorcluster, "Value"=w438:T23)  [unwired: 1 out]
                n74 = Unbundle By Name(w438) -> ("Start Position (N)"=w439:T17)
                n75 = Unbundle By Name(w438) -> ("Jump Position (m)"=w437:T17)
              }
              frame "none" {
                w443 = T13."Experiment Safe Position" ("Which Position to use for Experiment")
              }
            }
          }
          frame 3 {
            n76 = Unbundle By Name(w452) -> ("PhaseC Cluster"=w449:T15)
            n77 = Unbundle By Name(w449) -> ("Phase Experiment Option"=w451:refnum<vi>)
            n78 = property class="CmbBox"(reference=w451, error in=w446) -> (error out=w445:errorcluster, "Value"=w447:string)  [unwired: 1 out]
            n79 = case shown="\"Single Manip Jump\"" w447 {
              tunnel: w449 -> [_ w461 w467 w473 w480 w487 w494 w502 _]
              tunnel: [w454 w458 w465 w472 w479 w486 w493 w501 w505] -> w450
              tunnel: [w454 T13."Experiment Safe Position" ("Which Position to use for Experiment") T13."Experiment Safe Position" ("Which Position to use for Experiment") T13."Experiment Safe Position" ("Which Position to use for Experiment") T13."Experiment Safe Position" ("Which Position to use for Experiment") T13."Experiment Safe Position" ("Which Position to use for Experiment") T13."Experiment Safe Position" ("Which Position to use for Experiment") w499 w505] -> w448
              tunnel: w445 -> [w453 w456 w463 w470 w477 w484 w491 w498 w504]
              tunnel: [w453 w455 w462 w469 w476 w483 w490 w497 w504] -> w444
              frame "False", Default {
                w454 = T13."Experiment Safe Position" ("Which Position to use for Experiment")
              }
              frame "Single Jump" {
                n80 = Unbundle By Name(w461) -> ("Single Jump"=w460:refnum<vi>)
                n81 = property class="Clust (strict)"(reference=w460, error in=w456) -> (error out=w455:errorcluster, "Value"=w459:T16)  [unwired: 1 out]
                n82 = Unbundle By Name(w459) -> ("Which Position to use for Experiment"=w458:T17)
              }
              frame "Solution Change" {
                n83 = Unbundle By Name(w467) -> ("Solution Change"=w468:refnum<vi>)
                n84 = property class="Clust (strict)"(reference=w468, error in=w463) -> (error out=w462:errorcluster, "Value"=w466:T18)  [unwired: 1 out]
                n85 = Unbundle By Name(w466) -> ("Which Position to use for Experiment"=w465:T17)
              }
              frame "Voltage Step" {
                n86 = Unbundle By Name(w473) -> ("Voltage Step"=w475:refnum<vi>)
                n87 = property class="Clust (strict)"(reference=w475, error in=w470) -> (error out=w469:errorcluster, "Value"=w474:T19)  [unwired: 1 out]
                n88 = Unbundle By Name(w474) -> ("Which Position to use for Experiment"=w472:T17)
              }
              frame "Voltage Ramp" {
                n89 = Unbundle By Name(w480) -> ("Voltage Ramp"=w482:refnum<vi>)
                n90 = property class="Clust (strict)"(reference=w482, error in=w477) -> (error out=w476:errorcluster, "Value"=w481:T20)  [unwired: 1 out]
                n91 = Unbundle By Name(w481) -> ("Which Position to use for Experiment"=w479:T17)
              }
              frame "Jump Train" {
                n92 = Unbundle By Name(w487) -> ("Jump Train"=w489:refnum<vi>)
                n93 = property class="Clust (strict)"(reference=w489, error in=w484) -> (error out=w483:errorcluster, "Value"=w488:T21)  [unwired: 1 out]
                n94 = Unbundle By Name(w488) -> ("Which Position to use for Experiment"=w486:T17)
              }
              frame "Paired Pulse" {
                n95 = Unbundle By Name(w494) -> ("Paired Pulse"=w496:refnum<vi>)
                n96 = property class="Clust (strict)"(reference=w496, error in=w491) -> (error out=w490:errorcluster, "Value"=w495:T22)  [unwired: 1 out]
                n97 = Unbundle By Name(w495) -> ("Which Position to use for Experiment"=w493:T17)
              }
              frame "Single Manip Jump" {
                n98 = Unbundle By Name(w502) -> ("Single Manip Jump"=w503:refnum<vi>)
                n99 = property class="Clust (strict)"(reference=w503, error in=w498) -> (error out=w497:errorcluster, "Value"=w500:T23)  [unwired: 1 out]
                n100 = Unbundle By Name(w500) -> ("Start Position (N)"=w501:T17)
                n101 = Unbundle By Name(w500) -> ("Jump Position (m)"=w499:T17)
              }
              frame "none" {
                w505 = T13."Experiment Safe Position" ("Which Position to use for Experiment")
              }
            }
          }
          frame 4 {
            n102 = Unbundle By Name(w514) -> ("PhaseD Cluster"=w511:T15)
            n103 = Unbundle By Name(w511) -> ("Phase Experiment Option"=w513:refnum<vi>)
            n104 = property class="CmbBox"(reference=w513, error in=w508) -> (error out=w507:errorcluster, "Value"=w509:string)  [unwired: 1 out]
            n105 = case shown="\"Single Manip Jump\"" w509 {
              tunnel: w511 -> [_ w523 w529 w535 w542 w549 w556 w564 _]
              tunnel: [w516 w520 w527 w534 w541 w548 w555 w563 w567] -> w512
              tunnel: [w516 T13."Experiment Safe Position" ("Which Position to use for Experiment") T13."Experiment Safe Position" ("Which Position to use for Experiment") T13."Experiment Safe Position" ("Which Position to use for Experiment") T13."Experiment Safe Position" ("Which Position to use for Experiment") T13."Experiment Safe Position" ("Which Position to use for Experiment") T13."Experiment Safe Position" ("Which Position to use for Experiment") w561 w567] -> w510
              tunnel: w507 -> [w515 w518 w525 w532 w539 w546 w553 w560 w566]
              tunnel: [w515 w517 w524 w531 w538 w545 w552 w559 w566] -> w506
              frame "False", Default {
                w516 = T13."Experiment Safe Position" ("Which Position to use for Experiment")
              }
              frame "Single Jump" {
                n106 = Unbundle By Name(w523) -> ("Single Jump"=w522:refnum<vi>)
                n107 = property class="Clust (strict)"(reference=w522, error in=w518) -> (error out=w517:errorcluster, "Value"=w521:T16)  [unwired: 1 out]
                n108 = Unbundle By Name(w521) -> ("Which Position to use for Experiment"=w520:T17)
              }
              frame "Solution Change" {
                n109 = Unbundle By Name(w529) -> ("Solution Change"=w530:refnum<vi>)
                n110 = property class="Clust (strict)"(reference=w530, error in=w525) -> (error out=w524:errorcluster, "Value"=w528:T18)  [unwired: 1 out]
                n111 = Unbundle By Name(w528) -> ("Which Position to use for Experiment"=w527:T17)
              }
              frame "Voltage Step" {
                n112 = Unbundle By Name(w535) -> ("Voltage Step"=w537:refnum<vi>)
                n113 = property class="Clust (strict)"(reference=w537, error in=w532) -> (error out=w531:errorcluster, "Value"=w536:T19)  [unwired: 1 out]
                n114 = Unbundle By Name(w536) -> ("Which Position to use for Experiment"=w534:T17)
              }
              frame "Voltage Ramp" {
                n115 = Unbundle By Name(w542) -> ("Voltage Ramp"=w544:refnum<vi>)
                n116 = property class="Clust (strict)"(reference=w544, error in=w539) -> (error out=w538:errorcluster, "Value"=w543:T20)  [unwired: 1 out]
                n117 = Unbundle By Name(w543) -> ("Which Position to use for Experiment"=w541:T17)
              }
              frame "Jump Train" {
                n118 = Unbundle By Name(w549) -> ("Jump Train"=w551:refnum<vi>)
                n119 = property class="Clust (strict)"(reference=w551, error in=w546) -> (error out=w545:errorcluster, "Value"=w550:T21)  [unwired: 1 out]
                n120 = Unbundle By Name(w550) -> ("Which Position to use for Experiment"=w548:T17)
              }
              frame "Paired Pulse" {
                n121 = Unbundle By Name(w556) -> ("Paired Pulse"=w558:refnum<vi>)
                n122 = property class="Clust (strict)"(reference=w558, error in=w553) -> (error out=w552:errorcluster, "Value"=w557:T22)  [unwired: 1 out]
                n123 = Unbundle By Name(w557) -> ("Which Position to use for Experiment"=w555:T17)
              }
              frame "Single Manip Jump" {
                n124 = Unbundle By Name(w564) -> ("Single Manip Jump"=w565:refnum<vi>)
                n125 = property class="Clust (strict)"(reference=w565, error in=w560) -> (error out=w559:errorcluster, "Value"=w562:T23)  [unwired: 1 out]
                n126 = Unbundle By Name(w562) -> ("Start Position (N)"=w563:T17)
                n127 = Unbundle By Name(w562) -> ("Jump Position (m)"=w561:T17)
              }
              frame "none" {
                w567 = T13."Experiment Safe Position" ("Which Position to use for Experiment")
              }
            }
          }
          frame 5 {
            n128 = Unbundle By Name(w576) -> ("PhaseE Cluster"=w573:T15)
            n129 = Unbundle By Name(w573) -> ("Phase Experiment Option"=w575:refnum<vi>)
            n130 = property class="CmbBox"(reference=w575, error in=w570) -> (error out=w569:errorcluster, "Value"=w571:string)  [unwired: 1 out]
            n131 = case shown="\"Single Manip Jump\"" w571 {
              tunnel: w573 -> [_ w585 w591 w597 w604 w611 w618 w626 _]
              tunnel: [w578 w582 w589 w596 w603 w610 w617 w625 w629] -> w574
              tunnel: [w578 T13."Experiment Safe Position" ("Which Position to use for Experiment") T13."Experiment Safe Position" ("Which Position to use for Experiment") T13."Experiment Safe Position" ("Which Position to use for Experiment") T13."Experiment Safe Position" ("Which Position to use for Experiment") T13."Experiment Safe Position" ("Which Position to use for Experiment") T13."Experiment Safe Position" ("Which Position to use for Experiment") w623 w629] -> w572
              tunnel: w569 -> [w577 w580 w587 w594 w601 w608 w615 w622 w628]
              tunnel: [w577 w579 w586 w593 w600 w607 w614 w621 w628] -> w568
              frame "False", Default {
                w578 = T13."Experiment Safe Position" ("Which Position to use for Experiment")
              }
              frame "Single Jump" {
                n132 = Unbundle By Name(w585) -> ("Single Jump"=w584:refnum<vi>)
                n133 = property class="Clust (strict)"(reference=w584, error in=w580) -> (error out=w579:errorcluster, "Value"=w583:T16)  [unwired: 1 out]
                n134 = Unbundle By Name(w583) -> ("Which Position to use for Experiment"=w582:T17)
              }
              frame "Solution Change" {
                n135 = Unbundle By Name(w591) -> ("Solution Change"=w592:refnum<vi>)
                n136 = property class="Clust (strict)"(reference=w592, error in=w587) -> (error out=w586:errorcluster, "Value"=w590:T18)  [unwired: 1 out]
                n137 = Unbundle By Name(w590) -> ("Which Position to use for Experiment"=w589:T17)
              }
              frame "Voltage Step" {
                n138 = Unbundle By Name(w597) -> ("Voltage Step"=w599:refnum<vi>)
                n139 = property class="Clust (strict)"(reference=w599, error in=w594) -> (error out=w593:errorcluster, "Value"=w598:T19)  [unwired: 1 out]
                n140 = Unbundle By Name(w598) -> ("Which Position to use for Experiment"=w596:T17)
              }
              frame "Voltage Ramp" {
                n141 = Unbundle By Name(w604) -> ("Voltage Ramp"=w606:refnum<vi>)
                n142 = property class="Clust (strict)"(reference=w606, error in=w601) -> (error out=w600:errorcluster, "Value"=w605:T20)  [unwired: 1 out]
                n143 = Unbundle By Name(w605) -> ("Which Position to use for Experiment"=w603:T17)
              }
              frame "Jump Train" {
                n144 = Unbundle By Name(w611) -> ("Jump Train"=w613:refnum<vi>)
                n145 = property class="Clust (strict)"(reference=w613, error in=w608) -> (error out=w607:errorcluster, "Value"=w612:T21)  [unwired: 1 out]
                n146 = Unbundle By Name(w612) -> ("Which Position to use for Experiment"=w610:T17)
              }
              frame "Paired Pulse" {
                n147 = Unbundle By Name(w618) -> ("Paired Pulse"=w620:refnum<vi>)
                n148 = property class="Clust (strict)"(reference=w620, error in=w615) -> (error out=w614:errorcluster, "Value"=w619:T22)  [unwired: 1 out]
                n149 = Unbundle By Name(w619) -> ("Which Position to use for Experiment"=w617:T17)
              }
              frame "Single Manip Jump" {
                n150 = Unbundle By Name(w626) -> ("Single Manip Jump"=w627:refnum<vi>)
                n151 = property class="Clust (strict)"(reference=w627, error in=w622) -> (error out=w621:errorcluster, "Value"=w624:T23)  [unwired: 1 out]
                n152 = Unbundle By Name(w624) -> ("Start Position (N)"=w625:T17)
                n153 = Unbundle By Name(w624) -> ("Jump Position (m)"=w623:T17)
              }
              frame "none" {
                w629 = T13."Experiment Safe Position" ("Which Position to use for Experiment")
              }
            }
          }
          frame 6 {
            n154 = Unbundle By Name(w638) -> ("PhaseF Cluster"=w635:T15)
            n155 = Unbundle By Name(w635) -> ("Phase Experiment Option"=w637:refnum<vi>)
            n156 = property class="CmbBox"(reference=w637, error in=w632) -> (error out=w631:errorcluster, "Value"=w633:string)  [unwired: 1 out]
            n157 = case shown="\"Single Manip Jump\"" w633 {
              tunnel: w635 -> [_ w647 w653 w659 w666 w673 w680 w688 _]
              tunnel: [w640 w644 w651 w658 w665 w672 w679 w687 w691] -> w636
              tunnel: [w640 T13."Experiment Safe Position" ("Which Position to use for Experiment") T13."Experiment Safe Position" ("Which Position to use for Experiment") T13."Experiment Safe Position" ("Which Position to use for Experiment") T13."Experiment Safe Position" ("Which Position to use for Experiment") T13."Experiment Safe Position" ("Which Position to use for Experiment") T13."Experiment Safe Position" ("Which Position to use for Experiment") w685 w691] -> w634
              tunnel: w631 -> [w639 w642 w649 w656 w663 w670 w677 w684 w690]
              tunnel: [w639 w641 w648 w655 w662 w669 w676 w683 w690] -> w630
              frame "False", Default {
                w640 = T13."Experiment Safe Position" ("Which Position to use for Experiment")
              }
              frame "Single Jump" {
                n158 = Unbundle By Name(w647) -> ("Single Jump"=w646:refnum<vi>)
                n159 = property class="Clust (strict)"(reference=w646, error in=w642) -> (error out=w641:errorcluster, "Value"=w645:T16)  [unwired: 1 out]
                n160 = Unbundle By Name(w645) -> ("Which Position to use for Experiment"=w644:T17)
              }
              frame "Solution Change" {
                n161 = Unbundle By Name(w653) -> ("Solution Change"=w654:refnum<vi>)
                n162 = property class="Clust (strict)"(reference=w654, error in=w649) -> (error out=w648:errorcluster, "Value"=w652:T18)  [unwired: 1 out]
                n163 = Unbundle By Name(w652) -> ("Which Position to use for Experiment"=w651:T17)
              }
              frame "Voltage Step" {
                n164 = Unbundle By Name(w659) -> ("Voltage Step"=w661:refnum<vi>)
                n165 = property class="Clust (strict)"(reference=w661, error in=w656) -> (error out=w655:errorcluster, "Value"=w660:T19)  [unwired: 1 out]
                n166 = Unbundle By Name(w660) -> ("Which Position to use for Experiment"=w658:T17)
              }
              frame "Voltage Ramp" {
                n167 = Unbundle By Name(w666) -> ("Voltage Ramp"=w668:refnum<vi>)
                n168 = property class="Clust (strict)"(reference=w668, error in=w663) -> (error out=w662:errorcluster, "Value"=w667:T20)  [unwired: 1 out]
                n169 = Unbundle By Name(w667) -> ("Which Position to use for Experiment"=w665:T17)
              }
              frame "Jump Train" {
                n170 = Unbundle By Name(w673) -> ("Jump Train"=w675:refnum<vi>)
                n171 = property class="Clust (strict)"(reference=w675, error in=w670) -> (error out=w669:errorcluster, "Value"=w674:T21)  [unwired: 1 out]
                n172 = Unbundle By Name(w674) -> ("Which Position to use for Experiment"=w672:T17)
              }
              frame "Paired Pulse" {
                n173 = Unbundle By Name(w680) -> ("Paired Pulse"=w682:refnum<vi>)
                n174 = property class="Clust (strict)"(reference=w682, error in=w677) -> (error out=w676:errorcluster, "Value"=w681:T22)  [unwired: 1 out]
                n175 = Unbundle By Name(w681) -> ("Which Position to use for Experiment"=w679:T17)
              }
              frame "Single Manip Jump" {
                n176 = Unbundle By Name(w688) -> ("Single Manip Jump"=w689:refnum<vi>)
                n177 = property class="Clust (strict)"(reference=w689, error in=w684) -> (error out=w683:errorcluster, "Value"=w686:T23)  [unwired: 1 out]
                n178 = Unbundle By Name(w686) -> ("Start Position (N)"=w687:T17)
                n179 = Unbundle By Name(w686) -> ("Jump Position (m)"=w685:T17)
              }
              frame "none" {
                w691 = T13."Experiment Safe Position" ("Which Position to use for Experiment")
              }
            }
          }
          frame 7 {
            n180 = Unbundle By Name(w700) -> ("PhaseG Cluster"=w697:T15)
            n181 = Unbundle By Name(w697) -> ("Phase Experiment Option"=w699:refnum<vi>)
            n182 = property class="CmbBox"(reference=w699, error in=w694) -> (error out=w693:errorcluster, "Value"=w695:string)  [unwired: 1 out]
            n183 = case shown="\"Single Manip Jump\"" w695 {
              tunnel: w697 -> [_ w709 w715 w721 w728 w735 w742 w750 _]
              tunnel: [w702 w706 w713 w720 w727 w734 w741 w749 w753] -> w698
              tunnel: [w702 T13."Experiment Safe Position" ("Which Position to use for Experiment") T13."Experiment Safe Position" ("Which Position to use for Experiment") T13."Experiment Safe Position" ("Which Position to use for Experiment") T13."Experiment Safe Position" ("Which Position to use for Experiment") T13."Experiment Safe Position" ("Which Position to use for Experiment") T13."Experiment Safe Position" ("Which Position to use for Experiment") w747 w753] -> w696
              tunnel: w693 -> [w701 w704 w711 w718 w725 w732 w739 w746 w752]
              tunnel: [w701 w703 w710 w717 w724 w731 w738 w745 w752] -> w692
              frame "False", Default {
                w702 = T13."Experiment Safe Position" ("Which Position to use for Experiment")
              }
              frame "Single Jump" {
                n184 = Unbundle By Name(w709) -> ("Single Jump"=w708:refnum<vi>)
                n185 = property class="Clust (strict)"(reference=w708, error in=w704) -> (error out=w703:errorcluster, "Value"=w707:T16)  [unwired: 1 out]
                n186 = Unbundle By Name(w707) -> ("Which Position to use for Experiment"=w706:T17)
              }
              frame "Solution Change" {
                n187 = Unbundle By Name(w715) -> ("Solution Change"=w716:refnum<vi>)
                n188 = property class="Clust (strict)"(reference=w716, error in=w711) -> (error out=w710:errorcluster, "Value"=w714:T18)  [unwired: 1 out]
                n189 = Unbundle By Name(w714) -> ("Which Position to use for Experiment"=w713:T17)
              }
              frame "Voltage Step" {
                n190 = Unbundle By Name(w721) -> ("Voltage Step"=w723:refnum<vi>)
                n191 = property class="Clust (strict)"(reference=w723, error in=w718) -> (error out=w717:errorcluster, "Value"=w722:T19)  [unwired: 1 out]
                n192 = Unbundle By Name(w722) -> ("Which Position to use for Experiment"=w720:T17)
              }
              frame "Voltage Ramp" {
                n193 = Unbundle By Name(w728) -> ("Voltage Ramp"=w730:refnum<vi>)
                n194 = property class="Clust (strict)"(reference=w730, error in=w725) -> (error out=w724:errorcluster, "Value"=w729:T20)  [unwired: 1 out]
                n195 = Unbundle By Name(w729) -> ("Which Position to use for Experiment"=w727:T17)
              }
              frame "Jump Train" {
                n196 = Unbundle By Name(w735) -> ("Jump Train"=w737:refnum<vi>)
                n197 = property class="Clust (strict)"(reference=w737, error in=w732) -> (error out=w731:errorcluster, "Value"=w736:T21)  [unwired: 1 out]
                n198 = Unbundle By Name(w736) -> ("Which Position to use for Experiment"=w734:T17)
              }
              frame "Paired Pulse" {
                n199 = Unbundle By Name(w742) -> ("Paired Pulse"=w744:refnum<vi>)
                n200 = property class="Clust (strict)"(reference=w744, error in=w739) -> (error out=w738:errorcluster, "Value"=w743:T22)  [unwired: 1 out]
                n201 = Unbundle By Name(w743) -> ("Which Position to use for Experiment"=w741:T17)
              }
              frame "Single Manip Jump" {
                n202 = Unbundle By Name(w750) -> ("Single Manip Jump"=w751:refnum<vi>)
                n203 = property class="Clust (strict)"(reference=w751, error in=w746) -> (error out=w745:errorcluster, "Value"=w748:T23)  [unwired: 1 out]
                n204 = Unbundle By Name(w748) -> ("Start Position (N)"=w749:T17)
                n205 = Unbundle By Name(w748) -> ("Jump Position (m)"=w747:T17)
              }
              frame "none" {
                w753 = T13."Experiment Safe Position" ("Which Position to use for Experiment")
              }
            }
          }
          frame 8 {
            n206 = Unbundle By Name(w762) -> ("PhaseH Cluster"=w759:T15)
            n207 = Unbundle By Name(w759) -> ("Phase Experiment Option"=w761:refnum<vi>)
            n208 = property class="CmbBox"(reference=w761, error in=w756) -> (error out=w755:errorcluster, "Value"=w757:string)  [unwired: 1 out]
            n209 = case shown="\"Single Manip Jump\"" w757 {
              tunnel: w759 -> [_ w771 w777 w783 w790 w797 w804 w812 _]
              tunnel: [w764 w768 w775 w782 w789 w796 w803 w811 w815] -> w760
              tunnel: [w764 T13."Experiment Safe Position" ("Which Position to use for Experiment") T13."Experiment Safe Position" ("Which Position to use for Experiment") T13."Experiment Safe Position" ("Which Position to use for Experiment") T13."Experiment Safe Position" ("Which Position to use for Experiment") T13."Experiment Safe Position" ("Which Position to use for Experiment") T13."Experiment Safe Position" ("Which Position to use for Experiment") w809 w815] -> w758
              tunnel: w755 -> [w763 w766 w773 w780 w787 w794 w801 w808 w814]
              tunnel: [w763 w765 w772 w779 w786 w793 w800 w807 w814] -> w754
              frame "False", Default {
                w764 = T13."Experiment Safe Position" ("Which Position to use for Experiment")
              }
              frame "Single Jump" {
                n210 = Unbundle By Name(w771) -> ("Single Jump"=w770:refnum<vi>)
                n211 = property class="Clust (strict)"(reference=w770, error in=w766) -> (error out=w765:errorcluster, "Value"=w769:T16)  [unwired: 1 out]
                n212 = Unbundle By Name(w769) -> ("Which Position to use for Experiment"=w768:T17)
              }
              frame "Solution Change" {
                n213 = Unbundle By Name(w777) -> ("Solution Change"=w778:refnum<vi>)
                n214 = property class="Clust (strict)"(reference=w778, error in=w773) -> (error out=w772:errorcluster, "Value"=w776:T18)  [unwired: 1 out]
                n215 = Unbundle By Name(w776) -> ("Which Position to use for Experiment"=w775:T17)
              }
              frame "Voltage Step" {
                n216 = Unbundle By Name(w783) -> ("Voltage Step"=w785:refnum<vi>)
                n217 = property class="Clust (strict)"(reference=w785, error in=w780) -> (error out=w779:errorcluster, "Value"=w784:T19)  [unwired: 1 out]
                n218 = Unbundle By Name(w784) -> ("Which Position to use for Experiment"=w782:T17)
              }
              frame "Voltage Ramp" {
                n219 = Unbundle By Name(w790) -> ("Voltage Ramp"=w792:refnum<vi>)
                n220 = property class="Clust (strict)"(reference=w792, error in=w787) -> (error out=w786:errorcluster, "Value"=w791:T20)  [unwired: 1 out]
                n221 = Unbundle By Name(w791) -> ("Which Position to use for Experiment"=w789:T17)
              }
              frame "Jump Train" {
                n222 = Unbundle By Name(w797) -> ("Jump Train"=w799:refnum<vi>)
                n223 = property class="Clust (strict)"(reference=w799, error in=w794) -> (error out=w793:errorcluster, "Value"=w798:T21)  [unwired: 1 out]
                n224 = Unbundle By Name(w798) -> ("Which Position to use for Experiment"=w796:T17)
              }
              frame "Paired Pulse" {
                n225 = Unbundle By Name(w804) -> ("Paired Pulse"=w806:refnum<vi>)
                n226 = property class="Clust (strict)"(reference=w806, error in=w801) -> (error out=w800:errorcluster, "Value"=w805:T22)  [unwired: 1 out]
                n227 = Unbundle By Name(w805) -> ("Which Position to use for Experiment"=w803:T17)
              }
              frame "Single Manip Jump" {
                n228 = Unbundle By Name(w812) -> ("Single Manip Jump"=w813:refnum<vi>)
                n229 = property class="Clust (strict)"(reference=w813, error in=w808) -> (error out=w807:errorcluster, "Value"=w810:T23)  [unwired: 1 out]
                n230 = Unbundle By Name(w810) -> ("Start Position (N)"=w811:T17)
                n231 = Unbundle By Name(w810) -> ("Jump Position (m)"=w809:T17)
              }
              frame "none" {
                w815 = T13."Experiment Safe Position" ("Which Position to use for Experiment")
              }
            }
          }
          frame 9 {
            n232 = Unbundle By Name(w824) -> ("PhaseI Cluster"=w821:T15)
            n233 = Unbundle By Name(w821) -> ("Phase Experiment Option"=w823:refnum<vi>)
            n234 = property class="CmbBox"(reference=w823, error in=w818) -> (error out=w817:errorcluster, "Value"=w819:string)  [unwired: 1 out]
            n235 = case shown="\"Single Manip Jump\"" w819 {
              tunnel: w821 -> [_ w833 w839 w845 w852 w859 w866 w874 _]
              tunnel: [w826 w830 w837 w844 w851 w858 w865 w873 w877] -> w822
              tunnel: [w826 T13."Experiment Safe Position" ("Which Position to use for Experiment") T13."Experiment Safe Position" ("Which Position to use for Experiment") T13."Experiment Safe Position" ("Which Position to use for Experiment") T13."Experiment Safe Position" ("Which Position to use for Experiment") T13."Experiment Safe Position" ("Which Position to use for Experiment") T13."Experiment Safe Position" ("Which Position to use for Experiment") w871 w877] -> w820
              tunnel: w817 -> [w825 w828 w835 w842 w849 w856 w863 w870 w876]
              tunnel: [w825 w827 w834 w841 w848 w855 w862 w869 w876] -> w816
              frame "False", Default {
                w826 = T13."Experiment Safe Position" ("Which Position to use for Experiment")
              }
              frame "Single Jump" {
                n236 = Unbundle By Name(w833) -> ("Single Jump"=w832:refnum<vi>)
                n237 = property class="Clust (strict)"(reference=w832, error in=w828) -> (error out=w827:errorcluster, "Value"=w831:T16)  [unwired: 1 out]
                n238 = Unbundle By Name(w831) -> ("Which Position to use for Experiment"=w830:T17)
              }
              frame "Solution Change" {
                n239 = Unbundle By Name(w839) -> ("Solution Change"=w840:refnum<vi>)
                n240 = property class="Clust (strict)"(reference=w840, error in=w835) -> (error out=w834:errorcluster, "Value"=w838:T18)  [unwired: 1 out]
                n241 = Unbundle By Name(w838) -> ("Which Position to use for Experiment"=w837:T17)
              }
              frame "Voltage Step" {
                n242 = Unbundle By Name(w845) -> ("Voltage Step"=w847:refnum<vi>)
                n243 = property class="Clust (strict)"(reference=w847, error in=w842) -> (error out=w841:errorcluster, "Value"=w846:T19)  [unwired: 1 out]
                n244 = Unbundle By Name(w846) -> ("Which Position to use for Experiment"=w844:T17)
              }
              frame "Voltage Ramp" {
                n245 = Unbundle By Name(w852) -> ("Voltage Ramp"=w854:refnum<vi>)
                n246 = property class="Clust (strict)"(reference=w854, error in=w849) -> (error out=w848:errorcluster, "Value"=w853:T20)  [unwired: 1 out]
                n247 = Unbundle By Name(w853) -> ("Which Position to use for Experiment"=w851:T17)
              }
              frame "Jump Train" {
                n248 = Unbundle By Name(w859) -> ("Jump Train"=w861:refnum<vi>)
                n249 = property class="Clust (strict)"(reference=w861, error in=w856) -> (error out=w855:errorcluster, "Value"=w860:T21)  [unwired: 1 out]
                n250 = Unbundle By Name(w860) -> ("Which Position to use for Experiment"=w858:T17)
              }
              frame "Paired Pulse" {
                n251 = Unbundle By Name(w866) -> ("Paired Pulse"=w868:refnum<vi>)
                n252 = property class="Clust (strict)"(reference=w868, error in=w863) -> (error out=w862:errorcluster, "Value"=w867:T22)  [unwired: 1 out]
                n253 = Unbundle By Name(w867) -> ("Which Position to use for Experiment"=w865:T17)
              }
              frame "Single Manip Jump" {
                n254 = Unbundle By Name(w874) -> ("Single Manip Jump"=w875:refnum<vi>)
                n255 = property class="Clust (strict)"(reference=w875, error in=w870) -> (error out=w869:errorcluster, "Value"=w872:T23)  [unwired: 1 out]
                n256 = Unbundle By Name(w872) -> ("Start Position (N)"=w873:T17)
                n257 = Unbundle By Name(w872) -> ("Jump Position (m)"=w871:T17)
              }
              frame "none" {
                w877 = T13."Experiment Safe Position" ("Which Position to use for Experiment")
              }
            }
          }
          frame 10 {
            n258 = Unbundle By Name(w886) -> ("PhaseJ Cluster"=w883:T15)
            n259 = Unbundle By Name(w883) -> ("Phase Experiment Option"=w885:refnum<vi>)
            n260 = property class="CmbBox"(reference=w885, error in=w880) -> (error out=w879:errorcluster, "Value"=w881:string)  [unwired: 1 out]
            n261 = case shown="\"Single Manip Jump\"" w881 {
              tunnel: w883 -> [_ w895 w901 w907 w914 w921 w928 w936 _]
              tunnel: [w888 w892 w899 w906 w913 w920 w927 w935 w939] -> w884
              tunnel: [w888 T13."Experiment Safe Position" ("Which Position to use for Experiment") T13."Experiment Safe Position" ("Which Position to use for Experiment") T13."Experiment Safe Position" ("Which Position to use for Experiment") T13."Experiment Safe Position" ("Which Position to use for Experiment") T13."Experiment Safe Position" ("Which Position to use for Experiment") T13."Experiment Safe Position" ("Which Position to use for Experiment") w933 w939] -> w882
              tunnel: w879 -> [w887 w890 w897 w904 w911 w918 w925 w932 w938]
              tunnel: [w887 w889 w896 w903 w910 w917 w924 w931 w938] -> w878
              frame "False", Default {
                w888 = T13."Experiment Safe Position" ("Which Position to use for Experiment")
              }
              frame "Single Jump" {
                n262 = Unbundle By Name(w895) -> ("Single Jump"=w894:refnum<vi>)
                n263 = property class="Clust (strict)"(reference=w894, error in=w890) -> (error out=w889:errorcluster, "Value"=w893:T16)  [unwired: 1 out]
                n264 = Unbundle By Name(w893) -> ("Which Position to use for Experiment"=w892:T17)
              }
              frame "Solution Change" {
                n265 = Unbundle By Name(w901) -> ("Solution Change"=w902:refnum<vi>)
                n266 = property class="Clust (strict)"(reference=w902, error in=w897) -> (error out=w896:errorcluster, "Value"=w900:T18)  [unwired: 1 out]
                n267 = Unbundle By Name(w900) -> ("Which Position to use for Experiment"=w899:T17)
              }
              frame "Voltage Step" {
                n268 = Unbundle By Name(w907) -> ("Voltage Step"=w909:refnum<vi>)
                n269 = property class="Clust (strict)"(reference=w909, error in=w904) -> (error out=w903:errorcluster, "Value"=w908:T19)  [unwired: 1 out]
                n270 = Unbundle By Name(w908) -> ("Which Position to use for Experiment"=w906:T17)
              }
              frame "Voltage Ramp" {
                n271 = Unbundle By Name(w914) -> ("Voltage Ramp"=w916:refnum<vi>)
                n272 = property class="Clust (strict)"(reference=w916, error in=w911) -> (error out=w910:errorcluster, "Value"=w915:T20)  [unwired: 1 out]
                n273 = Unbundle By Name(w915) -> ("Which Position to use for Experiment"=w913:T17)
              }
              frame "Jump Train" {
                n274 = Unbundle By Name(w921) -> ("Jump Train"=w923:refnum<vi>)
                n275 = property class="Clust (strict)"(reference=w923, error in=w918) -> (error out=w917:errorcluster, "Value"=w922:T21)  [unwired: 1 out]
                n276 = Unbundle By Name(w922) -> ("Which Position to use for Experiment"=w920:T17)
              }
              frame "Paired Pulse" {
                n277 = Unbundle By Name(w928) -> ("Paired Pulse"=w930:refnum<vi>)
                n278 = property class="Clust (strict)"(reference=w930, error in=w925) -> (error out=w924:errorcluster, "Value"=w929:T22)  [unwired: 1 out]
                n279 = Unbundle By Name(w929) -> ("Which Position to use for Experiment"=w927:T17)
              }
              frame "Single Manip Jump" {
                n280 = Unbundle By Name(w936) -> ("Single Manip Jump"=w937:refnum<vi>)
                n281 = property class="Clust (strict)"(reference=w937, error in=w932) -> (error out=w931:errorcluster, "Value"=w934:T23)  [unwired: 1 out]
                n282 = Unbundle By Name(w934) -> ("Start Position (N)"=w935:T17)
                n283 = Unbundle By Name(w934) -> ("Jump Position (m)"=w933:T17)
              }
              frame "none" {
                w939 = T13."Experiment Safe Position" ("Which Position to use for Experiment")
              }
            }
          }
          frame 11 {
            n284 = Unbundle By Name(w948) -> ("PhaseK Cluster"=w945:T15)
            n285 = Unbundle By Name(w945) -> ("Phase Experiment Option"=w947:refnum<vi>)
            n286 = property class="CmbBox"(reference=w947, error in=w942) -> (error out=w941:errorcluster, "Value"=w943:string)  [unwired: 1 out]
            n287 = case shown="\"Single Manip Jump\"" w943 {
              tunnel: w945 -> [_ w957 w963 w969 w976 w983 w990 w998 _]
              tunnel: [w950 w954 w961 w968 w975 w982 w989 w997 w1001] -> w946
              tunnel: [w950 T13."Experiment Safe Position" ("Which Position to use for Experiment") T13."Experiment Safe Position" ("Which Position to use for Experiment") T13."Experiment Safe Position" ("Which Position to use for Experiment") T13."Experiment Safe Position" ("Which Position to use for Experiment") T13."Experiment Safe Position" ("Which Position to use for Experiment") T13."Experiment Safe Position" ("Which Position to use for Experiment") w995 w1001] -> w944
              tunnel: w941 -> [w949 w952 w959 w966 w973 w980 w987 w994 w1000]
              tunnel: [w949 w951 w958 w965 w972 w979 w986 w993 w1000] -> w940
              frame "False", Default {
                w950 = T13."Experiment Safe Position" ("Which Position to use for Experiment")
              }
              frame "Single Jump" {
                n288 = Unbundle By Name(w957) -> ("Single Jump"=w956:refnum<vi>)
                n289 = property class="Clust (strict)"(reference=w956, error in=w952) -> (error out=w951:errorcluster, "Value"=w955:T16)  [unwired: 1 out]
                n290 = Unbundle By Name(w955) -> ("Which Position to use for Experiment"=w954:T17)
              }
              frame "Solution Change" {
                n291 = Unbundle By Name(w963) -> ("Solution Change"=w964:refnum<vi>)
                n292 = property class="Clust (strict)"(reference=w964, error in=w959) -> (error out=w958:errorcluster, "Value"=w962:T18)  [unwired: 1 out]
                n293 = Unbundle By Name(w962) -> ("Which Position to use for Experiment"=w961:T17)
              }
              frame "Voltage Step" {
                n294 = Unbundle By Name(w969) -> ("Voltage Step"=w971:refnum<vi>)
                n295 = property class="Clust (strict)"(reference=w971, error in=w966) -> (error out=w965:errorcluster, "Value"=w970:T19)  [unwired: 1 out]
                n296 = Unbundle By Name(w970) -> ("Which Position to use for Experiment"=w968:T17)
              }
              frame "Voltage Ramp" {
                n297 = Unbundle By Name(w976) -> ("Voltage Ramp"=w978:refnum<vi>)
                n298 = property class="Clust (strict)"(reference=w978, error in=w973) -> (error out=w972:errorcluster, "Value"=w977:T20)  [unwired: 1 out]
                n299 = Unbundle By Name(w977) -> ("Which Position to use for Experiment"=w975:T17)
              }
              frame "Jump Train" {
                n300 = Unbundle By Name(w983) -> ("Jump Train"=w985:refnum<vi>)
                n301 = property class="Clust (strict)"(reference=w985, error in=w980) -> (error out=w979:errorcluster, "Value"=w984:T21)  [unwired: 1 out]
                n302 = Unbundle By Name(w984) -> ("Which Position to use for Experiment"=w982:T17)
              }
              frame "Paired Pulse" {
                n303 = Unbundle By Name(w990) -> ("Paired Pulse"=w992:refnum<vi>)
                n304 = property class="Clust (strict)"(reference=w992, error in=w987) -> (error out=w986:errorcluster, "Value"=w991:T22)  [unwired: 1 out]
                n305 = Unbundle By Name(w991) -> ("Which Position to use for Experiment"=w989:T17)
              }
              frame "Single Manip Jump" {
                n306 = Unbundle By Name(w998) -> ("Single Manip Jump"=w999:refnum<vi>)
                n307 = property class="Clust (strict)"(reference=w999, error in=w994) -> (error out=w993:errorcluster, "Value"=w996:T23)  [unwired: 1 out]
                n308 = Unbundle By Name(w996) -> ("Start Position (N)"=w997:T17)
                n309 = Unbundle By Name(w996) -> ("Jump Position (m)"=w995:T17)
              }
              frame "none" {
                w1001 = T13."Experiment Safe Position" ("Which Position to use for Experiment")
              }
            }
          }
          frame 12 {
            n310 = Unbundle By Name(w1010) -> ("PhaseL Cluster"=w1007:T15)
            n311 = Unbundle By Name(w1007) -> ("Phase Experiment Option"=w1009:refnum<vi>)
            n312 = property class="CmbBox"(reference=w1009, error in=w1004) -> (error out=w1003:errorcluster, "Value"=w1005:string)  [unwired: 1 out]
            n313 = case shown="\"Voltage Ramp\"" w1005 {
              tunnel: w1007 -> [_ w1019 w1025 w1031 w1038 w1045 w1052 w1060 _]
              tunnel: [w1012 w1016 w1023 w1030 w1037 w1044 w1051 w1059 w1063] -> w1008
              tunnel: [w1012 T13."Experiment Safe Position" ("Which Position to use for Experiment") T13."Experiment Safe Position" ("Which Position to use for Experiment") T13."Experiment Safe Position" ("Which Position to use for Experiment") T13."Experiment Safe Position" ("Which Position to use for Experiment") T13."Experiment Safe Position" ("Which Position to use for Experiment") T13."Experiment Safe Position" ("Which Position to use for Experiment") w1057 w1063] -> w1006
              tunnel: w1003 -> [w1011 w1014 w1021 w1028 w1035 w1042 w1049 w1056 w1062]
              tunnel: [w1011 w1013 w1020 w1027 w1034 w1041 w1048 w1055 w1062] -> w1002
              frame "False", Default {
                w1012 = T13."Experiment Safe Position" ("Which Position to use for Experiment")
              }
              frame "Single Jump" {
                n314 = Unbundle By Name(w1019) -> ("Single Jump"=w1018:refnum<vi>)
                n315 = property class="Clust (strict)"(reference=w1018, error in=w1014) -> (error out=w1013:errorcluster, "Value"=w1017:T16)  [unwired: 1 out]
                n316 = Unbundle By Name(w1017) -> ("Which Position to use for Experiment"=w1016:T17)
              }
              frame "Solution Change" {
                n317 = Unbundle By Name(w1025) -> ("Solution Change"=w1026:refnum<vi>)
                n318 = property class="Clust (strict)"(reference=w1026, error in=w1021) -> (error out=w1020:errorcluster, "Value"=w1024:T18)  [unwired: 1 out]
                n319 = Unbundle By Name(w1024) -> ("Which Position to use for Experiment"=w1023:T17)
              }
              frame "Voltage Step" {
                n320 = Unbundle By Name(w1031) -> ("Voltage Step"=w1033:refnum<vi>)
                n321 = property class="Clust (strict)"(reference=w1033, error in=w1028) -> (error out=w1027:errorcluster, "Value"=w1032:T19)  [unwired: 1 out]
                n322 = Unbundle By Name(w1032) -> ("Which Position to use for Experiment"=w1030:T17)
              }
              frame "Voltage Ramp" {
                n323 = Unbundle By Name(w1038) -> ("Voltage Ramp"=w1040:refnum<vi>)
                n324 = property class="Clust (strict)"(reference=w1040, error in=w1035) -> (error out=w1034:errorcluster, "Value"=w1039:T20)  [unwired: 1 out]
                n325 = Unbundle By Name(w1039) -> ("Which Position to use for Experiment"=w1037:T17)
              }
              frame "Jump Train" {
                n326 = Unbundle By Name(w1045) -> ("Jump Train"=w1047:refnum<vi>)
                n327 = property class="Clust (strict)"(reference=w1047, error in=w1042) -> (error out=w1041:errorcluster, "Value"=w1046:T21)  [unwired: 1 out]
                n328 = Unbundle By Name(w1046) -> ("Which Position to use for Experiment"=w1044:T17)
              }
              frame "Paired Pulse" {
                n329 = Unbundle By Name(w1052) -> ("Paired Pulse"=w1054:refnum<vi>)
                n330 = property class="Clust (strict)"(reference=w1054, error in=w1049) -> (error out=w1048:errorcluster, "Value"=w1053:T22)  [unwired: 1 out]
                n331 = Unbundle By Name(w1053) -> ("Which Position to use for Experiment"=w1051:T17)
              }
              frame "Single Manip Jump" {
                n332 = Unbundle By Name(w1060) -> ("Single Manip Jump"=w1061:refnum<vi>)
                n333 = property class="Clust (strict)"(reference=w1061, error in=w1056) -> (error out=w1055:errorcluster, "Value"=w1058:T23)  [unwired: 1 out]
                n334 = Unbundle By Name(w1058) -> ("Start Position (N)"=w1059:T17)
                n335 = Unbundle By Name(w1058) -> ("Jump Position (m)"=w1057:T17)
              }
              frame "none" {
                w1063 = T13."Experiment Safe Position" ("Which Position to use for Experiment")
              }
            }
          }
        }
        n336 = Equal?(x=w146, y="Single Manip Jump") -> (x = y?=w144:bool)
        n337 = case shown="False" w144 {
          tunnel: w128 -> [w188 w266]
          tunnel: w151 -> [w187 w279]
          tunnel: w150 -> [w186 w278]
          tunnel: w149 -> [w185 w280]
          tunnel: w148 -> [w184 w277]
          tunnel: w147 -> [w183 w281]
          tunnel: w127 -> [_ w265]
          tunnel: [w181 w276] -> w142
          tunnel: [w180 w275] -> w126
          tunnel: [w179 w274] -> w125
          tunnel: w137 -> [w178 w269]
          tunnel: [w176 w273] -> w136
          tunnel: w131 -> [w175 w272]
          tunnel: w130 -> [w174 _]
          tunnel: w129 -> [w173 w271]
          tunnel: [w171 w270] -> w124
          tunnel: [w169 w260] -> w120
          tunnel: w109 -> [_ w268]
          tunnel: w108 -> [_ w267]
          frame False {
            n338 = case shown="\"Jumper Position A\"" w188 {
              tunnel: [w235 w237 w239 w241 w243 w245 w247 w249 w251 w253 w255 w257 w259] -> w170
              tunnel: [w234 w236 w238 w240 w242 w244 w246 w248 w250 w252 w254 w256 w258] -> w189
              frame "Jumper Safe Position", Default {
                n339 = local read "Jumper Safe"() -> (w235:bool)
                n340 = control-ref of="Jumper Safe"() -> (w234:refnum<vi>)
              }
              frame "Experiment Safe Position" {
                n341 = local read "Experiment Safe"() -> (w237:bool)
                n342 = control-ref of="Experiment Safe"() -> (w236:refnum<vi>)
              }
              frame "Jumper Position A" {
                n343 = local read "Pos A"() -> (w239:bool)
                n344 = control-ref of="Pos A"() -> (w238:refnum<vi>)
              }
              frame "Jumper Position B" {
                n345 = local read "Pos B"() -> (w241:bool)
                n346 = control-ref of="Pos B"() -> (w240:refnum<vi>)
              }
              frame "Jumper Position C" {
                n347 = local read "Pos C"() -> (w243:bool)
                n348 = control-ref of="Pos C"() -> (w242:refnum<vi>)
              }
              frame "Jumper Position o-A" {
                n349 = control-ref of="Jump Pos o-A"() -> (w244:refnum<vi>)
                n350 = local read "Jump Pos o-A"() -> (w245:bool)
              }
              frame "Jumper Position A-o" {
                n351 = local read "Jump Pos A-o"() -> (w247:bool)
                n352 = control-ref of="Jump Pos A-o"() -> (w246:refnum<vi>)
              }
              frame "Jumper Position A-B" {
                n353 = local read "Jump Pos A-B"() -> (w249:bool)
                n354 = control-ref of="Jump Pos A-B"() -> (w248:refnum<vi>)
              }
              frame "Jumper Position B-A" {
                n355 = local read "Jump Pos B-A"() -> (w251:bool)
                n356 = control-ref of="Jump Pos B-A"() -> (w250:refnum<vi>)
              }
              frame "Jumper Position B-C" {
                n357 = control-ref of="Jump Pos B-C"() -> (w252:refnum<vi>)
                n358 = local read "Jump Pos B-C"() -> (w253:bool)
              }
              frame "Jumper Position C-B" {
                n359 = local read "Jump Pos C-B"() -> (w255:bool)
                n360 = control-ref of="Jump Pos C-B"() -> (w254:refnum<vi>)
              }
              frame "Jumper Position C-o" {
                n361 = control-ref of="Jump Pos C-o"() -> (w256:refnum<vi>)
                n362 = local read "Jump Pos C-o"() -> (w257:bool)
              }
              frame "Jumper Position o-C" {
                n363 = control-ref of="Jump Pos o-C"() -> (w258:refnum<vi>)
                n364 = local read "Jump Pos o-C"() -> (w259:bool)
              }
            }
            n365 = flat-sequence {
              tunnel: w170 -> [w205]
              tunnel: w188 -> [w204]
              tunnel: w187 -> [w203]
              tunnel: w186 -> [w202]
              tunnel: w185 -> [w201]
              tunnel: w184 -> [w200]
              tunnel: w183 -> [w199]
              tunnel: [w198] -> w182
              tunnel: [w197] -> w180
              tunnel: [w196] -> w179
              tunnel: w178 -> [w195]
              tunnel: [w194] -> w177
              tunnel: w175 -> [w193]
              tunnel: w174 -> [w192]
              tunnel: w173 -> [w191]
              tunnel: [w190] -> w172
              tunnel: w189 -> [w233]
              tunnel: [w231] -> w181
              tunnel: w182 -> [w231]
              tunnel: w177 -> [w230]
              tunnel: [w230] -> w176
              tunnel: [w229] -> w171
              tunnel: w172 -> [w229]
              frame #0 {
                n366 = case shown="False" w205 {
                  tunnel: w204 -> [w217 _]
                  tunnel: w203 -> [w219 _]
                  tunnel: w202 -> [w218 _]
                  tunnel: w201 -> [w216 _]
                  tunnel: w200 -> [w215 _]
                  tunnel: w199 -> [w214 w228]
                  tunnel: [w213 w228] -> w198
                  tunnel: [w212 w221] -> w197
                  tunnel: [w211 w223] -> w196
                  tunnel: w195 -> [w210 w227]
                  tunnel: [w209 w227] -> w194
                  tunnel: w193 -> [w208 _]
                  tunnel: w192 -> [_ w226]
                  tunnel: w191 -> [w207 _]
                  tunnel: [w206 T12 {"daq_ao 2"="", "Duration (s)"=0.0, "Sample Freq (Hz)"=0.0, "Phase"=0.0, "Duty Cycle"=0.0, "Jump Filter Freq (Hz)"=0.0, "Number of Replicates"=0} ("output cluster")] -> w190
                  frame False {
                    n367 = call "validate_position_v0.01.vi"("valve Time Cluster"=w207, "which manipulator"=w216, "Which Position to use for Experiment"=w217, "data in"=w215, "controls array in"=w214, "time to wait for solution change (min)"=w208, "error in"=w210, "common cluster"=w219, "individual controls in"=w218) -> ("output cluster"=w206:T12, "output waveform"=w212:waveform(dbl), "protocol response"=w211:waveform(dbl)[], "control array out"=w213:refnum<vi>[], "error out"=w209:errorcluster)  [unwired: 2 in]
                  }
                  frame True {
                    n368 = Unbundle By Name(w226) -> ("Command steps (mV)"=w225:refnum<vi>, "Recorded currents (pA)"=w224:refnum<vi>)
                    n369 = property class="WFGraph (strict)"(reference=w224) -> ("Value"=w223:waveform(dbl)[])  [unwired: 1 in, 2 out]
                    n370 = property class="WFGraph (strict)"(reference=w225) -> ("Value"=w222:waveform(dbl)[])  [unwired: 1 in, 2 out]
                    n371 = Index Array(array=w222) -> (element=w221:waveform(dbl))  [unwired: 1 in]
                  }
                }
              }
              frame #1 {
                n372 = property class="Bool (strict)"(reference=w233, "Value"=TRUE) -> ()  [unwired: 1 in, 2 out]
              }
            }
            n373 = Not(x=w170) -> (.not. x?=w169:bool)
          }
          frame True {
            n374 = flat-sequence {
              tunnel: w269 -> [w301]
              tunnel: [w301] -> w264
              tunnel: w268 -> [w304]
              tunnel: w267 -> [w303]
              tunnel: w266 -> [w307]
              tunnel: w265 -> [w306]
              tunnel: [w305] -> w263
              tunnel: w264 -> [w305]
              frame #0 {
                "curMJumpAlreadyValid" <- FALSE ("curMJumpAlreadyValid")
              }
              frame #1 {
                n375 = Array Size(array=w304) -> (size(s)=w308:i32)
                n376 = for {
                  N: w308 -> [_]
                  tunnel: w307 -> [w315]
                  tunnel: w306 -> [w314]
                  tunnel: w304 -> [w310] mode=indexing
                  tunnel: w303 -> [w309] mode=indexing
                  n377 = Equal?(x=w310, y=w315) -> (x = y?=w313:bool)
                  n378 = Equal?(x=w309, y=w314) -> (x = y?=w312:bool)
                  n379 = And(x=w313, y=w312) -> (x .and. y?=w311:bool)
                  n380 = case shown="True" w311 {
                    selector: w311 -> [_ w316]
                    frame False {
                    }
                    frame True {
                      n381 = local write "curMJumpAlreadyValid"(w316) -> ()
                    }
                  }
                }
              }
            }
            n382 = local read "curMJumpAlreadyValid"() -> (w262:bool)
            n383 = case shown="False" w262 {
              selector: w262 -> [w282 w298]
              tunnel: w281 -> [w297 w299]
              tunnel: w280 -> [w296 _]
              tunnel: w279 -> [w295 _]
              tunnel: w278 -> [w294 _]
              tunnel: w277 -> [w293 _]
              tunnel: [w292 w299] -> w276
              tunnel: [w291 _] -> w275
              tunnel: [w290 _] -> w274
              tunnel: [w289 w300] -> w273
              tunnel: w272 -> [w288 _]
              tunnel: w271 -> [w287 _]
              tunnel: [w286 _] -> w270
              tunnel: w266 -> [w285 _]
              tunnel: w265 -> [w284 _]
              tunnel: w263 -> [w283 w300]
              tunnel: [w282 w298] -> w261
              frame False {
                n384 = call "validate_ManipJump_v0.01.vi"("Start Position"=w285, "which manipulator"=w296, "valve Time Cluster"=w287, "data in"=w293, "Jump Position"=w284, "controls array in"=w297, "time to wait for solution change (min)"=w288, "error in"=w283, "common cluster"=w295, "individual controls in"=w294) -> ("output cluster"=w286:T12, "protocol waveform"=w291:waveform(dbl), "protocol response"=w290:waveform(dbl)[], "control array out"=w292:refnum<vi>[], "error out"=w289:errorcluster)  [unwired: 1 in]
              }
              frame True {
              }
            }
            n385 = Not(x=w261) -> (.not. x?=w260:bool)
          }
        }
        "protocol waveform" <- w126
        "protocol response" <- w125
        n386 = Unbundle By Name(w130) -> ("Command steps (mV)"=w141:refnum<vi>, "Recorded currents (pA)"=w140:refnum<vi>)
        n387 = Build Array(w126) -> (w139:waveform(dbl)[])
        n388 = call "Time Delay2"("error in (no error)"=w136) -> ("error out"=w135:errorcluster)  [unwired: 10 in]
        n389 = property class="WFGraph (strict)"(reference=w140, error in=w135, "Value"=w125) -> (error out=w134:errorcluster)  [unwired: 1 out]
        n390 = property class="WFGraph (strict)"(reference=w141, error in=w135, "Value"=w139) -> (error out=w132:errorcluster)  [unwired: 1 out]
        n391 = Build Array (concatenate)(w108, w127) -> (w118:T24)
        n392 = Build Array (concatenate)(w123, w124) -> (w116:T2)
        n393 = Build Array (concatenate)(w109, w128) -> (w119:T24)
        n394 = Build Array (concatenate)(w122, w126) -> (w117:waveform(dbl)[])
        n395 = Build Array (concatenate)(w121, w125) -> (w115:waveform(dbl)[][])
        n396 = case shown="False" w120 {
          tunnel: w119 -> [w163 w168]
          tunnel: w118 -> [w161 w167]
          tunnel: w117 -> [w159 w166]
          tunnel: w116 -> [w157 w165]
          tunnel: w115 -> [w155 w164]
          tunnel: [w162 w168] -> w114
          tunnel: [w160 w167] -> w113
          tunnel: [w158 w166] -> w112
          tunnel: [w156 w165] -> w111
          tunnel: [w154 w164] -> w110
          frame False {
            n397 = Delete From Array(array=w161) -> (array with subset deleted=w160:T24)  [unwired: 2 in, 1 out]
            n398 = Delete From Array(array=w163) -> (array with subset deleted=w162:T24)  [unwired: 2 in, 1 out]
            n399 = Delete From Array(array=w157) -> (array with subset deleted=w156:T2)  [unwired: 2 in, 1 out]
            n400 = Delete From Array(array=w155) -> (array with subset deleted=w154:waveform(dbl)[][])  [unwired: 3 in, 1 out]
            n401 = Delete From Array(array=w159) -> (array with subset deleted=w158:waveform(dbl)[])  [unwired: 2 in, 1 out]
          }
          frame True {
          }
        }
        n402 = Merge Errors(w132, w134) -> (w133:errorcluster)
      }
      "ValidationPos1" <- w91
      "ValidationPos2" <- w90
      "ValidationWaveform" <- w89
      "ValidationResults" <- w88
      "ValidationOutputCluster" <- w87
    }
    frame #2 {
      w1075 = u16 1 ("ChangeToValve")
      w1076 = TRUE ("Set Status")
      # "valve 2"
      # "valve 1"
      n403 = Unbundle By Name(w1074) -> ("misc indiv.daq_do 1"=w1073:tag, "misc indiv.daq_do 2"=w1072:tag, "misc indiv.V1-State"=w1071:refnum<vi>, "misc indiv.V2-State"=w1070:refnum<vi>)
      n404 = call "setPressure_topLvl.vi"("which manipulator"=w1083, "Slide Refnum"=w1084, "error in"=w1081, "set pressure (mBar)"=0.0, "Pressure box control in"=w1082) -> ("error out"=w1080:errorcluster)  [unwired: 5 in, 1 out]
      n405 = property class="DigNum (strict)"(reference=w1071) -> (reference out=w1069:refnum<vi>, "Value"=w1067:u16)  [unwired: 1 in, 1 out]
      n406 = call "sendValveSignal-v02.2.vi"("daq_do"=w1073, "Valve1?"=w1076, "ChangeToValve"=w1075, "CurrentValve"=w1067, "controls array in"=w1078, "Set Status"=w1076) -> ("ValveSetTo"=w1065:u16, "control array out"=w1079:refnum<vi>[])  [unwired: 6 in, 2 out]
      n407 = property class="DigNum (strict)"(reference=w1070) -> (reference out=w1068:refnum<vi>, "Value"=w1066:u16)  [unwired: 1 in, 1 out]
      n408 = call "sendValveSignal-v02.2.vi"("daq_do"=w1072, "ChangeToValve"=w1075, "CurrentValve"=w1066, "controls array in"=w1079, "Set Status"=w1076) -> ("ValveSetTo"=w1064:u16, "control array out"=w1077:refnum<vi>[])  [unwired: 7 in, 2 out]
    }
    frame #3 {
      n409 = property class="DigNum (strict)"(reference=w1089, "Value"=w1087) -> ()  [unwired: 1 in, 2 out]
      n410 = property class="DigNum (strict)"(reference=w1088, "Value"=w1086) -> ()  [unwired: 1 in, 2 out]
    }
  }
  n411 = Request Deallocation(TRUE ("flag")) -> ()
  "error out" <- w39
  "Experiment Safe" <- w20
  "Pos A" <- w20
  "Pos B" <- w20
  "Pos C" <- w20
  "Jump Pos o-A" <- w18
  "Jump Pos A-o" <- w18
  "Jump Pos A-B" <- w18
  "Jump Pos B-A" <- w18
  "Jump Pos B-C" <- w18
  "Jump Pos C-B" <- w18
  "Jump Pos C-o" <- w18
  "Jumper Safe" <- w20
  "Jump Pos o-C" <- w18
  "control array out" <- w17
